vi "Code Compare Tool For Git.vi"() -> ()   [LabVIEW 2016]
doc: "GUI to compare LabVIEW code between currently checked out branch with any other branch or any of its commits"
uses:
  <vilib>/Hampel Software Engineering/Git API/Git API/GIT-api.lvclass
  <vilib>/Hampel Software Engineering/Git API/Git API/GIT-api.lvclass/GIT-api.ctl
  <vilib>/Hampel Software Engineering/Git API/Git API/Controls/GIT-Repository States.ctl
  <vilib>/Utility/miscctls.llb/LVComboBoxStrsAndValuesArrayTypeDef.ctl
  <vilib>/Hampel Software Engineering/Git API/Git API/Accessors/GIT-Set Working Dir.vi
  <userlib>/_OpenG.lib/file/file.llb/Valid Path - Traditional__ogtk.vi
  <userlib>/_OpenG.lib/file/file.llb/File Exists - Scalar__ogtk.vi
  <userlib>/_OpenG.lib/array/array.llb/Delete Elements from 2D Array (String)__ogtk.vi
  <userlib>/_OpenG.lib/array/array.llb/Remove Duplicates from 1D Array (String)__ogtk.vi
  <userlib>/_OpenG.lib/array/array.llb/Search 1D Array (String)__ogtk.vi
  <userlib>/_OpenG.lib/array/array.llb/Remove Duplicates from 1D Array (Path)__ogtk.vi
panel:
  in  "Tab Control":T1(tab)=enum."Main UI"
  in  "All Files Selection":enum8{"False", "True", "Mixed"}(c332)
  in  "Refresh Current Branch":bool
  in  "Commits to Fetch":u32=10 min=1 step=10
  out "No Changes":bool
  in  "Compare Mode":enum32{"With Branch", "With Commit"}(radio)
  out "Commit Details":string
  in  "Commit":string(combo) caption="Recent Commit"
  in  "Stop":bool
  in  "Repository Path":path
  out "Current Branch":string
  in  "Branch":string(combo)="origin/main" caption="Branch to Compare"
  in  "Current Branch Changelist":i32(listbox)=-1
  in  "LabVIEW Compare Filter":bool
  out "Changelist Stats":string
  in  "Compare":bool
  out "Current Branch Status":string
  out "Current Branch Highlight":bool=TRUE
  out "Branch Highlight":bool=TRUE
  out "Commit Highlight":bool
  in  "LabVIEW Compare Options":T2={"VI Attributes"=TRUE, "Front Panel"=TRUE, "FP position/size"=TRUE, "Block Diagram"=TRUE, "BD cosmetic"=TRUE, "BD position/size"=TRUE}
  # "GUI to compare LabVIEW code between currently checked out branch with any other branch or any of its commits.\n\n\n1. Checkout the branch of interest in your system using any method - Git command line, Desktop Git GUI Clients etc.,\n\n2. Specify the local Repository Path.\n\n3. Verify the current branch, its status and select a branch or commit based on the Compare Mode and click on Compare to display the file changes.\n\n4. Double click on a file to initiate LabVIEW code comparison.\n\n5. Once done with required comparisons, exit the tool by closing the window. The tool cleans up the temporary files added during comparison.\n\n\nNote:\n1. This tool uses LabVIEW's VI Comparison Tool which requires LabVIEW Professional Development System.\n2. It is recommended to not use other Git Clients actively when comparing files using this tool to avoid Git command related errors.\n3. It is recommended to commit all changes (working copy) before using this tool for comparison."
  # "This tool uses git diff command to identify the changes. Hence it is recommended to commit all the changes (working copy) to have them considered for comparison.\n\nExample: Identify changes in current branch when comparing with other branch\n\n---A---B---C---D    <== other branch\n               \\\n                 E---F      <== current branch\n\n1. We will need to identify only the file changes introduced by current branch. E and F commits are those changes in the above example (commits after the common ancestor B).\n2. For the identified file changes compare with the other branch (D) to see how it differs. These differences will be our current branch changelist.\n\nWhy only current branch changes?\nIt is most useful to see how the current branch will modify the files when it is getting merged. Best use case for displaying only current branch changelist will be for Pull Request reviews."
  # "*Double click on modified LabVIEW file row to compare\n*Ctrl+Double click on a row to open file"
  # "Type Info:\n \nA - Added                     D - Deleted\nC* - Copied                  R* - Renamed\nM - Modified               T - File type change\nU - File is unmerged   X -  \"unknown\" change type\n\n*Number after C/R indicates the percentage of similarity between original and copied/renamed file"
  # "1. Repository Path - Local repository path (the top level folder with '.git' hidden folder in it). Git API will be initialized for this repository.\n\n2. Current Branch - Currently checked out branch. The status of the current branch is also displayed at top right. Click Refresh button to update the current branch if it is changed in the system or received new changes via Git Pull.\n\n3. Compare Mode - Select the type of comparison. You can compare the current branch with another branch or with a particular commit of a selected branch.\n\nIn branch comparison mode, you can enter the branch name for comparison in Branch to Compare. Remote branches usually start with \"origin/\" and local branches do not have \"origin/\" prefix. The branch's recent commit is displayed in Recent Commit and its details in Commit Details for reference. \n\nIn commit comparison mode, the commits available in the branch selected in Select Branch are listed in Commit to Compare. For the commit selected in Commit to Compare, its details will be displayed in the Commit Details. Use Commits to Fetch to limit the number of commits obtained and improve the loading time.\n\n     Note: Git doesn't maintain information on when the branch is created. So, all the commits of the selected branch will be displayed (all the way up to the very first commit after repository creation). Without a limit, it increases loading time.\n\n4. Compare - Identifies the file changes and Current Branch Changelist table shows the list of all files that are different in the current branch compared to the branch/commit selected.\n\n     Note: The other branch/commit in comparison would have introduced its own changes that are not part of current branch. Those changes will not be displayed.\n\n5. Filter LabVIEW VI and Control Files - Filter files except VI and CTL files. These require LabVIEW to compare but project, library and classes are text files that can be easily reviewed in the desktop Git GUI clients or in Pull Request of Git web services.\n\n6. LabVIEW Compare Options - Options to decide what to compare in the code. Set the required options before initiating code compare.\n\n7. Double click on the file you wish to compare. LabVIEW opens the compare window for the file from the current branch and the file from the other branch/commit (file will be suffixed with TEMP). It may take a while if the VI/CTL have lot of dependencies to load. Having the project pre-opened and opening this tool from that instance may reduce the loading time. Note that the file from the other branch/commit in comparison may be missing its dependent files which may not be available in the current branch or deleted in the current branch commits. This will cause the file to be in a broken state but does not affect the comparison. Another reason for the broken state may be due to the parent library/class not recognizing this new file with the suffix but this as well will not affect the comparison.\n\n     Note: The files from other branch/commit are placed at the same location in the current branch so that the LabVIEW can load the dependencies appropriately.\n\n8. Viewed Status (mixed checkbox) - A tick mark appears for every file compared or opened. Use the mixed checkbox (below the Current Branch Changelist) to control status for all files.\n\n     Note: Viewed status is only a visual aid for tracking and does not have any other function other than that.\n\n9. Panel Close - Stops the tools execution after removing all the new files introduced into the current branch (TEMP files)."
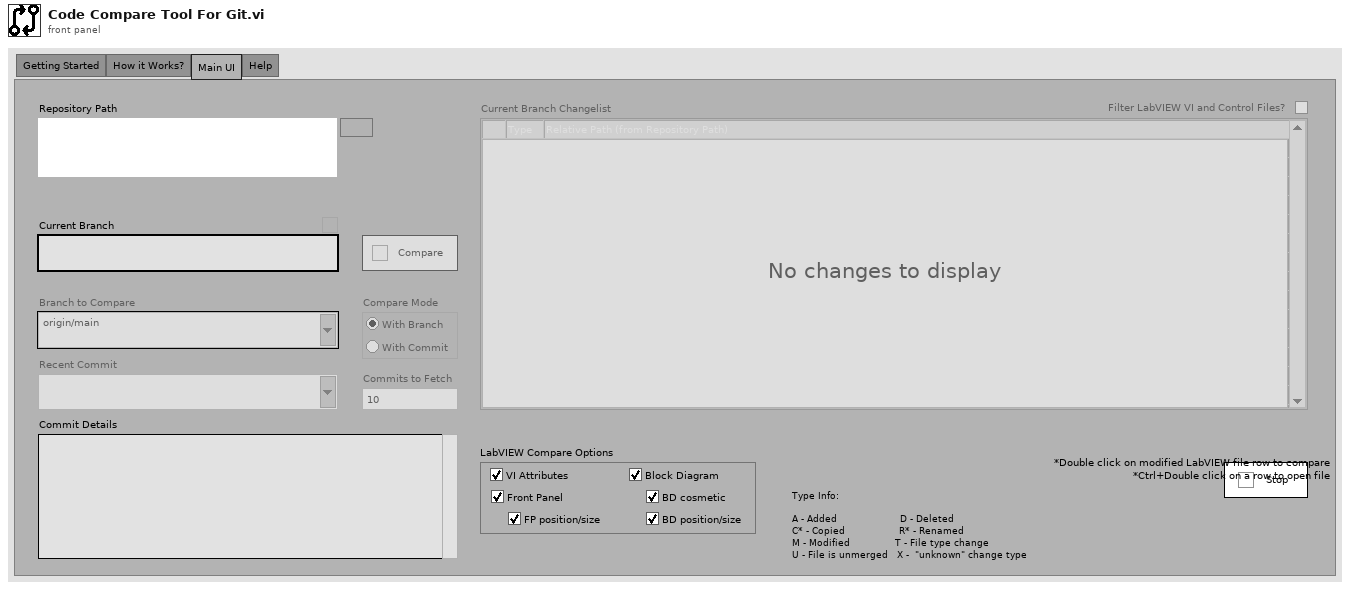
[diagram p1: front panel]
types:
  T1 = enum32{"Getting Started", "How it Works?", "Main UI", "Help"}
  T2 = cluster{"VI Attributes":bool, "Front Panel":bool, "FP position/size":bool, "Block Diagram":bool, "BD cosmetic":bool, "BD position/size":bool}
  T3 = cluster{"Repository Path":path, "Git API Object":refnum<class "GIT-api.lvclass">, "Git API Initialized?":bool, "Current Branch":string, "Compare Mode":enum32{"With Branch", "With Commit"}, "Branch to Compare":string, "Commit to Compare":string, "Commits to Fetch":u32, "Branch/Commit to Compare":string, "Changelist":string[][], "Viewed Files":string[], "Viewed File":string, "LabVIEW Compare Filter":bool, "LabVIEW Compare File Extensions":string[], "File to Open":string, "File to Compare":string, "File to Compare (backup)":path, "File to Compare (other)":path, "LabVIEW Compare Options":cluster{"VI Attributes":bool, "Front Panel":bool, "FP position/size":bool, "Block Diagram":bool, "BD cosmetic":bool, "BD position/size":bool}, "LabVIEW Compare Options Command":string, "Files to Delete":path[]}
  T4 = enum8{"Enabled", "Disabled", "Disabled and Grayed Out"}
  T5 = typedef "GIT-API-for-LabVIEW.lvlib/GIT-api.lvclass/GIT-Repository States.ctl" = enum16{"up-to-date", "behind", "ahead", "diverged", "unpublished", "detached", "unknown"}
  T6 = typedef "LVComboBoxStrsAndValuesArrayTypeDef.ctl" = cluster{"String":string, "Value":string}[]
  T7 = typedef "LVPoint32TypeDef.ctl" = cluster{"Horizontal":i32, "Vertical":i32}
  T8 = typedef "LVRowAndColumnTypeDef.ctl" = cluster{"Row":i32, "Column":i32}
  T9 = enum16{"Left Button", "Center Button", "Right Button", "Window Close"}
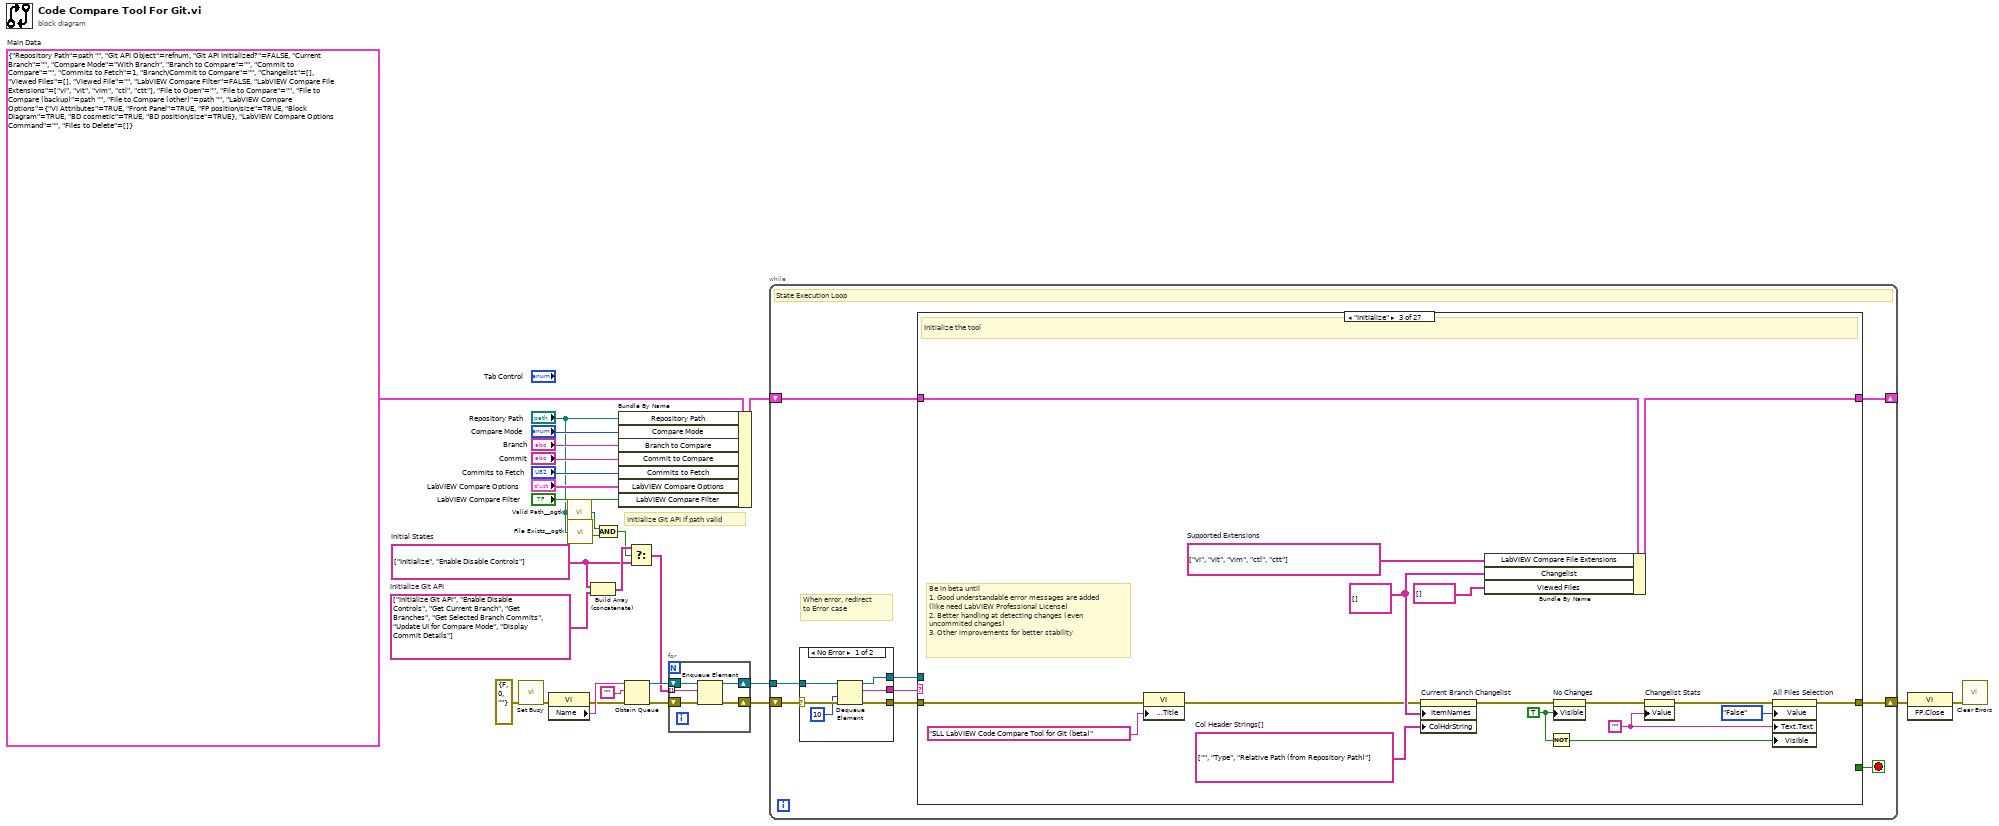
[diagram p0: block diagram]
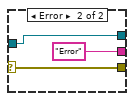
[diagram p2: hidden frame]
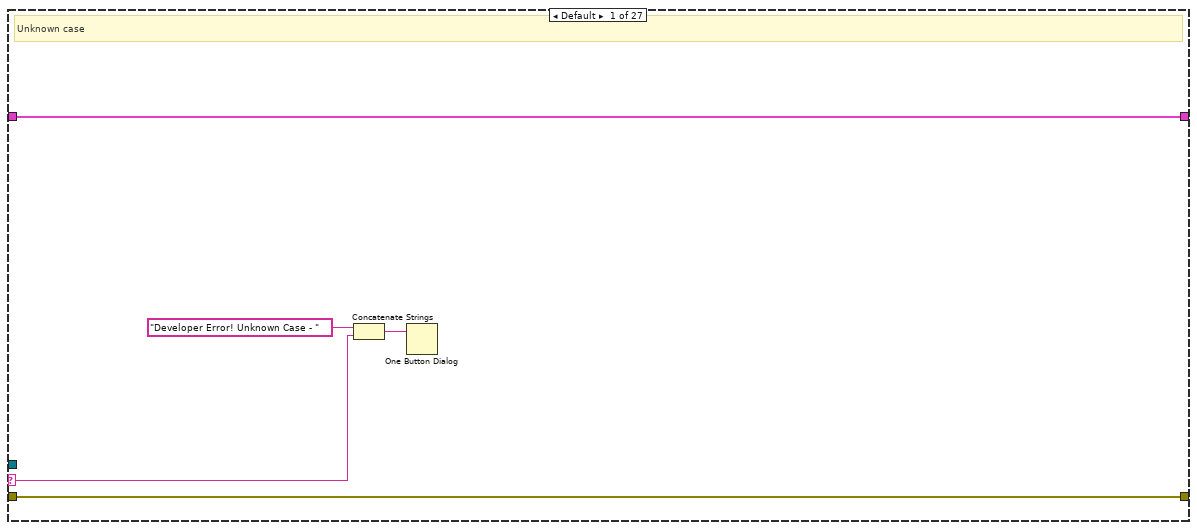
[diagram p3: hidden frame]
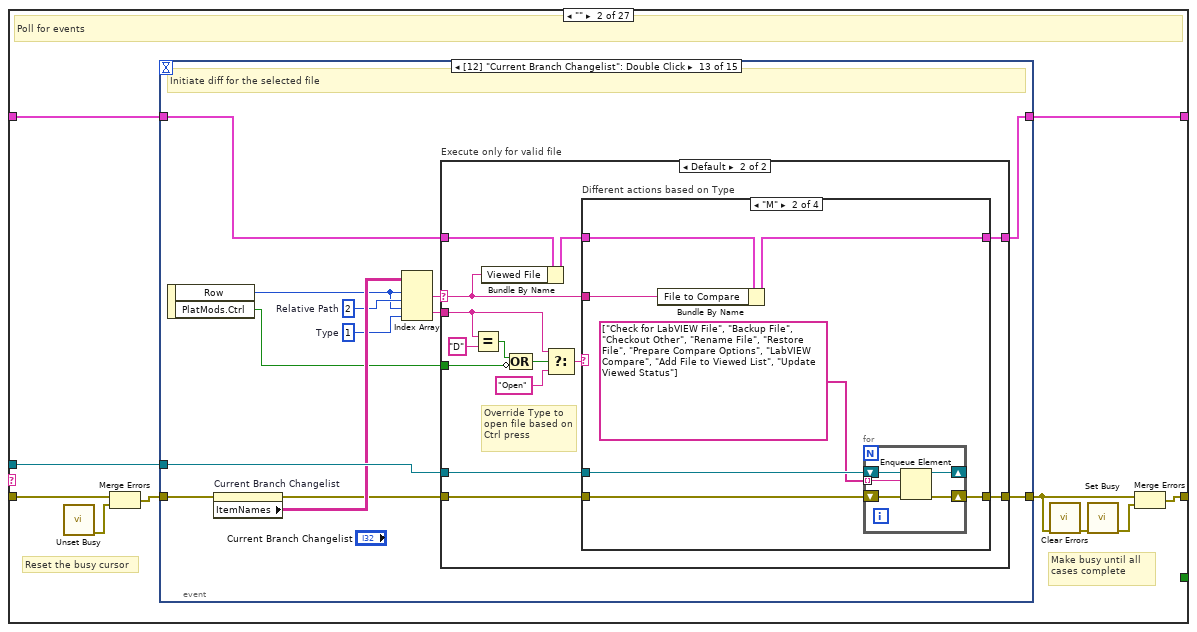
[diagram p4: hidden frame]
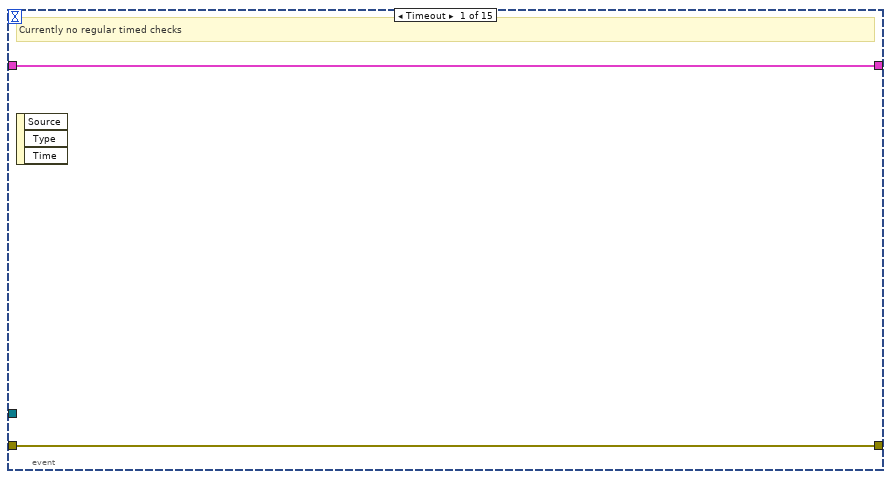
[diagram p5: hidden frame]
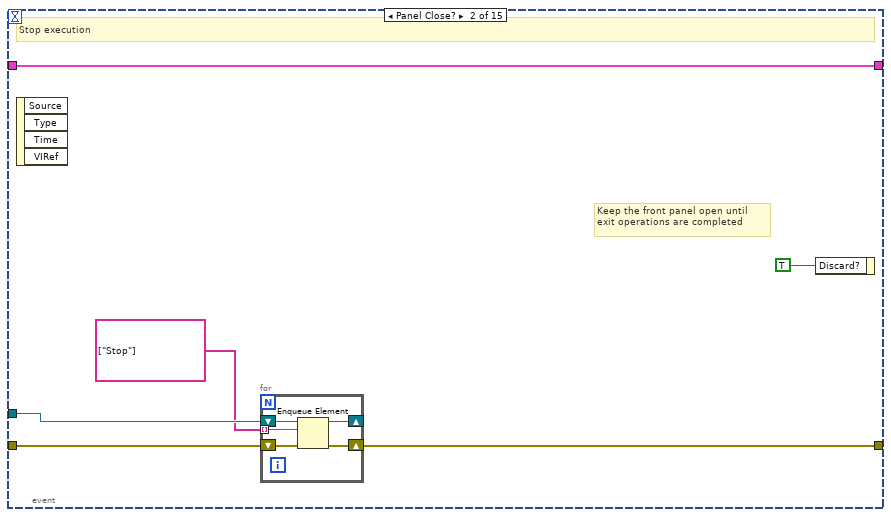
[diagram p6: hidden frame]
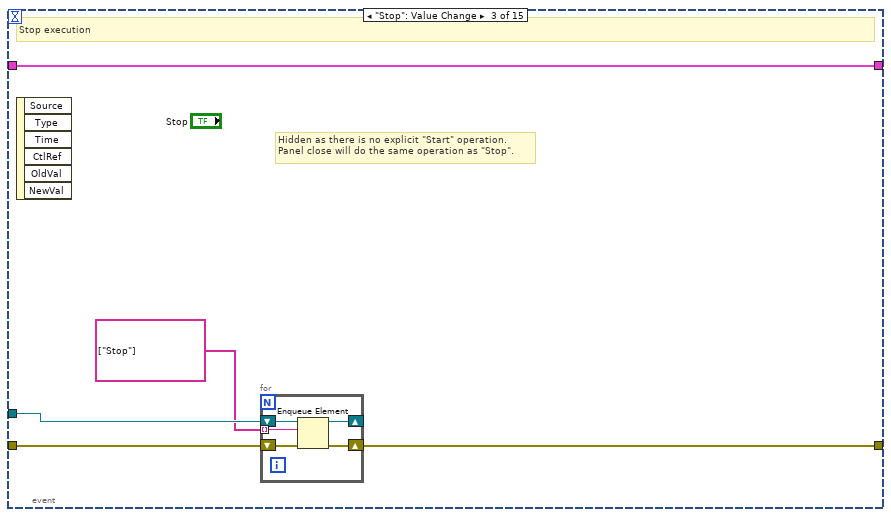
[diagram p7: hidden frame]
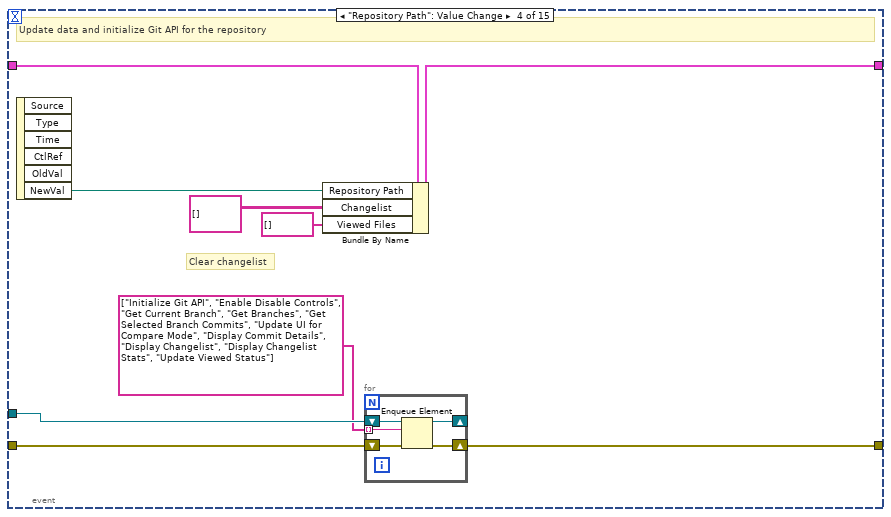
[diagram p8: hidden frame]
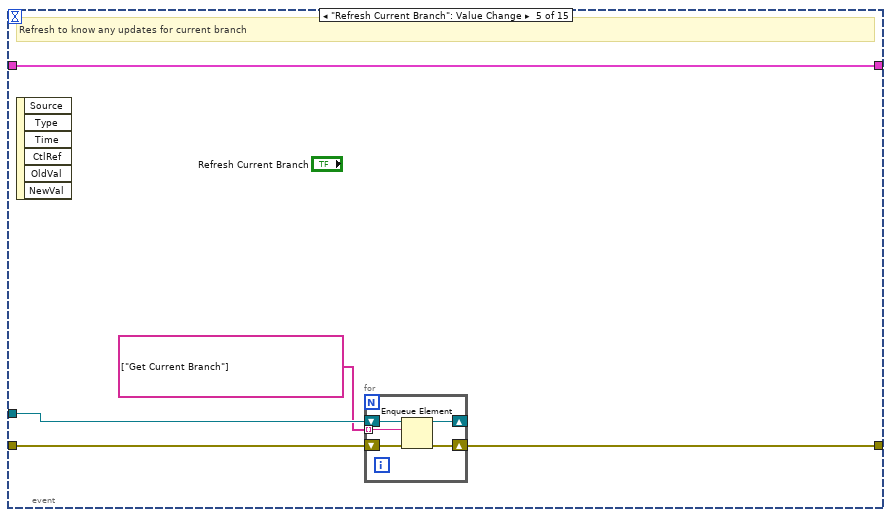
[diagram p9: hidden frame]
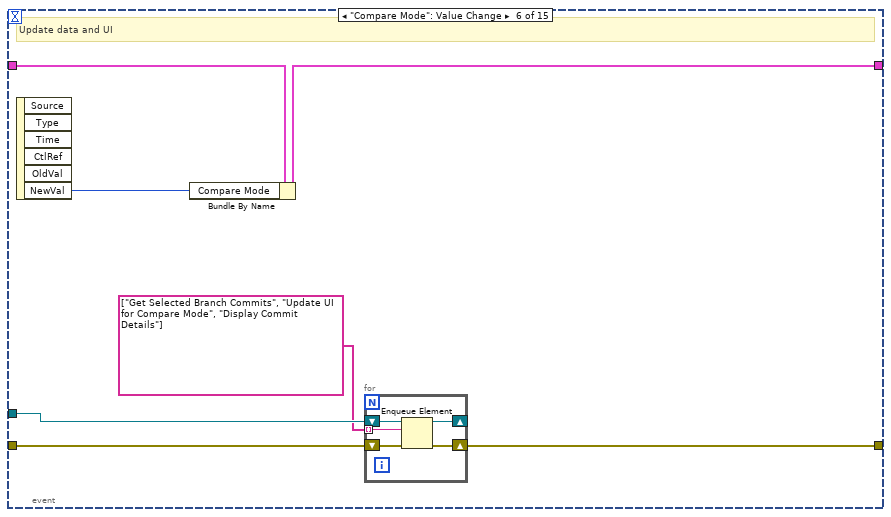
[diagram p10: hidden frame]
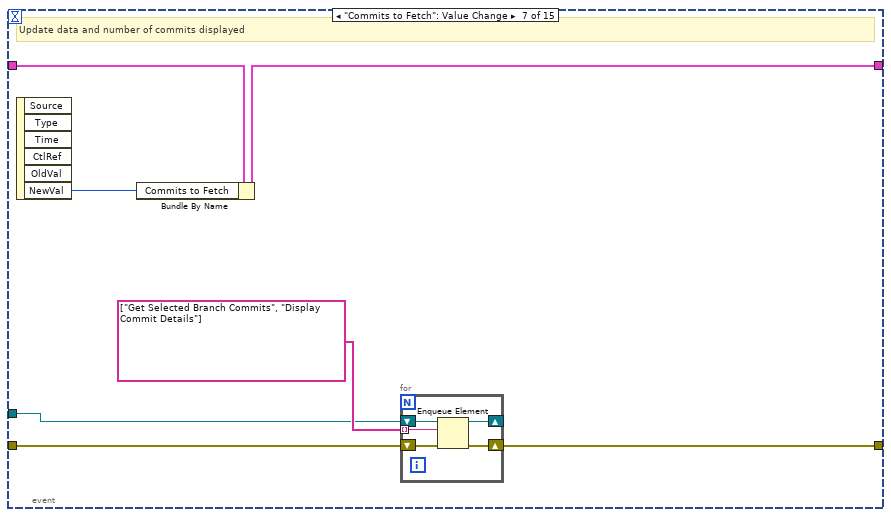
[diagram p11: hidden frame]
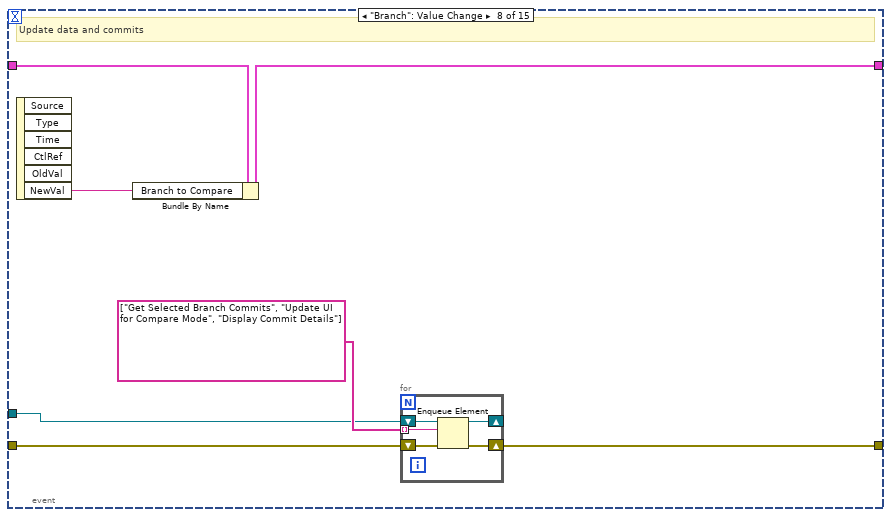
[diagram p12: hidden frame]
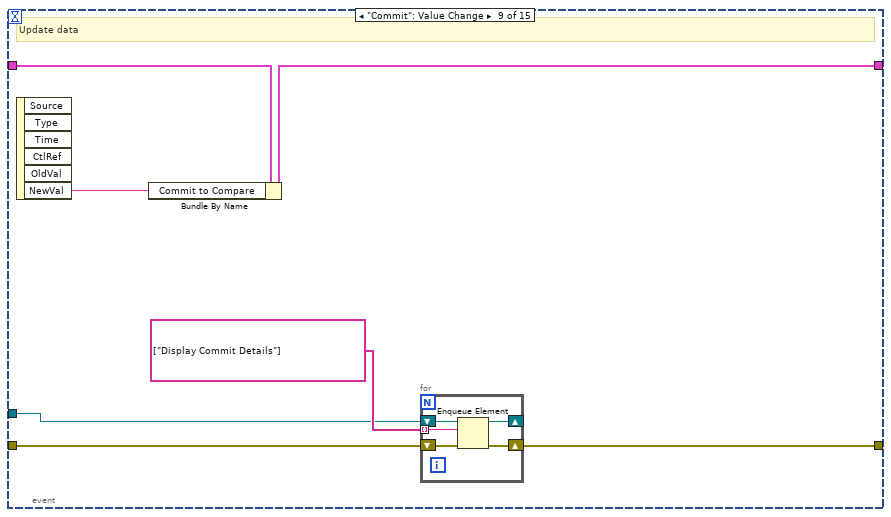
[diagram p13: hidden frame]
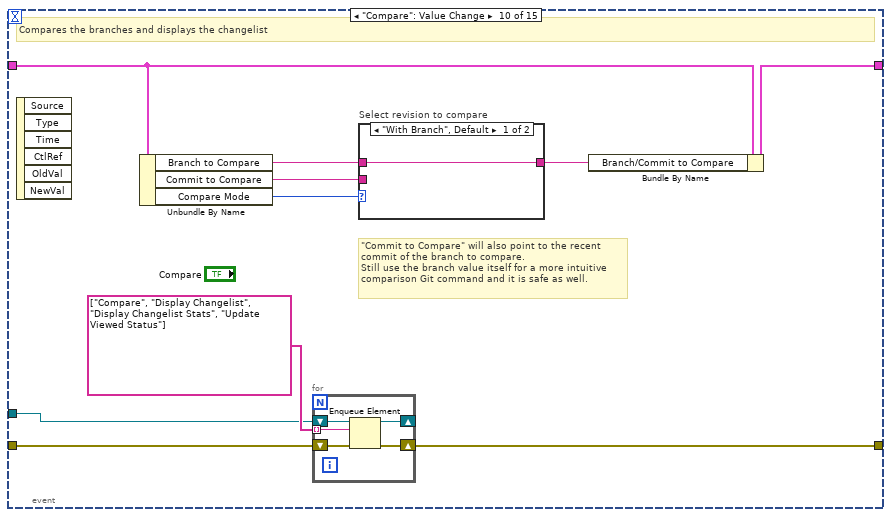
[diagram p14: hidden frame]
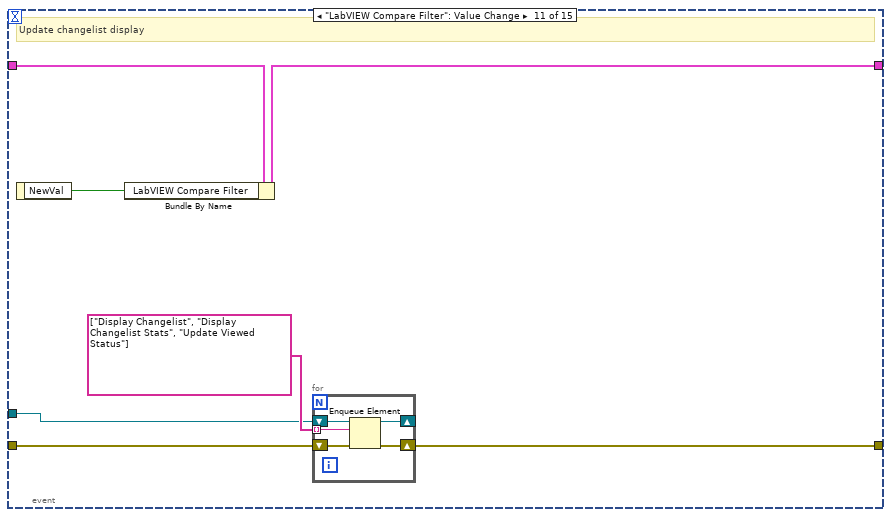
[diagram p16: hidden frame]
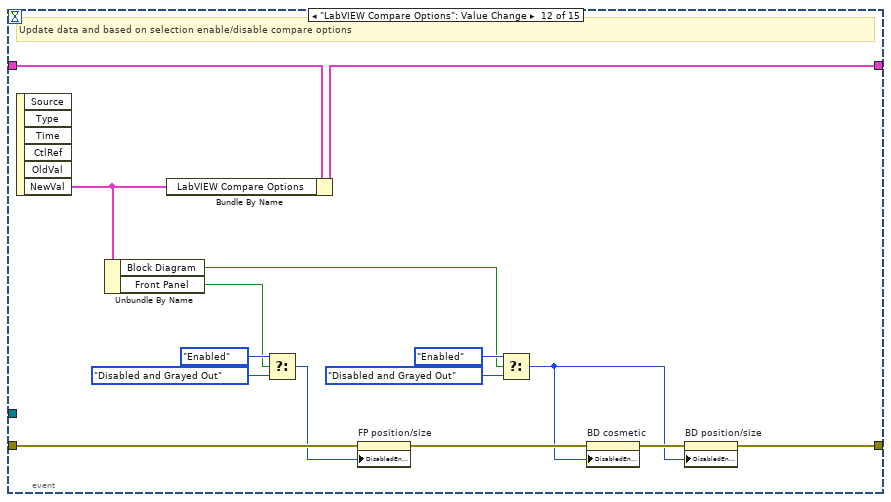
[diagram p17: hidden frame]
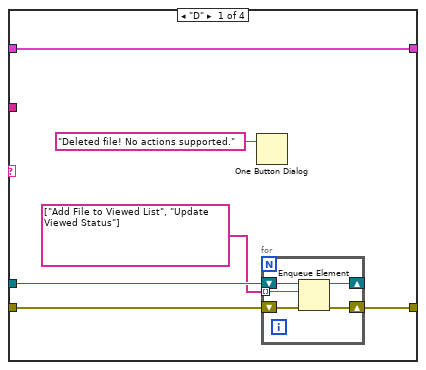
[diagram p19: hidden frame]
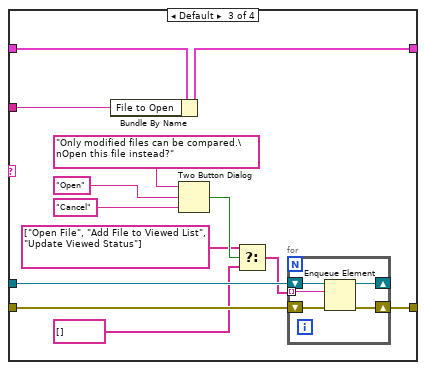
[diagram p20: hidden frame]
diagram:
  w16 = string[] ["Initialize Git API", "Enable Disable Controls", "Get Current Branch", "Get Branches", "Get Selected Branch Commits", "Update UI for Compare Mode", "Display Commit Details"]  # Initialize Git API
  w14 = string[] ["Initialize", "Enable Disable Controls"]  # Initial States
  w24 = T3 {"Repository Path"=path "", "Git API Object"=refnum, "Git API Initialized?"=FALSE, "Current Branch"="", "Compare Mode"=enum."With Branch", "Branch to Compare"="", "Commit to Compare"="", "Commits to Fetch"=1, "Branch/Commit to Compare"="", "Changelist"=[], "Viewed Files"=[], "Viewed File"="", "LabVIEW Compare Filter"=FALSE, "LabVIEW Compare File Extensions"=["vi", "vit", "vim", "ctl", "ctt"], "File to Open"="", "File to Compare"="", "File to Compare (backup)"=path "", "File to Compare (other)"=path "", "LabVIEW Compare Options"={"VI Attributes"=TRUE, "Front Panel"=TRUE, "FP position/size"=TRUE, "Block Diagram"=TRUE, "BD cosmetic"=TRUE, "BD position/size"=TRUE}, "LabVIEW Compare Options Command"="", "Files to Delete"=[]}  # Main Data
  # "Initialize Git API if path valid"
  n1 = call <vilib>:"Set Busy.vi"("error in (no error)"=errorcluster {"status"=FALSE, "code"=0, "source"=""}) -> ("error out"=w7:errorcluster)  [unwired: 9 in, 1 out]
  n2 = property class="VI"(error in=w7) -> (error out=w26:errorcluster, "Name"=w27:string)  [unwired: 1 in, 1 out]
  n3 = call-poly <userlib>:"Valid Path__ogtk.vi"("path"="Repository Path") -> ("valid"=w11:bool)
  n4 = call-poly <userlib>:"File Exists__ogtk.vi"("file path"="Repository Path") -> ("exists"=w12:bool)  [unwired: 6 in, 1 out]
  n5 = Build Array (concatenate)(w14, w16) -> (w15:string[])
  n6 = And(x=w11, y=w12) -> (x .and. y?=w10:bool)
  n7 = Bundle By Name(cluster=w24, "Repository Path"="Repository Path", "Compare Mode"="Compare Mode", "Branch to Compare"="Branch", "Commit to Compare"="Commit", "Commits to Fetch"="Commits to Fetch", "LabVIEW Compare Options"="LabVIEW Compare Options", "LabVIEW Compare Filter"="LabVIEW Compare Filter") -> (w23:T3)
  n8 = Obtain Queue(name (unnamed)=w27, element data type="", error in (no error)=w26) -> (queue out=w20:refnum<queue>, error out=w17:errorcluster)  [unwired: 2 in, 1 out]
  n9 = Select(t=w15, s=w10, f=w14) -> (s? t:f=w13:string[])
  n10 = for {
    tunnel: w13 -> [w29] mode=indexing
    shift-right: [w31] -> w19
    shift-left: w17 -> [w32]
    shift-right: [w28] -> w18
    shift-left: w20 -> [w30]
    n11 = Enqueue Element(queue=w30, element=w29, error in (no error)=w32) -> (queue out=w28:refnum<queue>, error out=w31:errorcluster)  [unwired: 1 in, 1 out]
  }
  n12 = while {
    shift-right: [w33] -> w2
    shift-left: w19 -> [w35]
    tunnel: w18 -> [w36]
    shift-right: [w38] -> _
    shift-left: w23 -> [w37]
    stop <- w39 stop-if-true
    # "When error, redirect to Error case"
    # "State Execution Loop"
    n13 = case shown="No Error" w35 {
      selector: w35 -> [w44 w48]
      tunnel: [w47 "Error" ("element")] -> w41
      tunnel: [w46 w50] -> w40
      tunnel: w36 -> [w45 w50]
      tunnel: [w42 w48] -> w34
      frame No Error {
        n14 = Dequeue Element(queue=w45, timeout in ms (-1)=10, error in (no error)=w44) -> (queue out=w46:refnum<queue>, element=w47:string, error out=w42:errorcluster)  [unwired: 1 out]
      }
      frame Error {
      }
    }
    n15 = case shown="\"Initialize\"" w41 {
      selector: w41 -> [w54 _ _ _ _ _ _ _ _ _ _ _ _ _ _ _ _ _ _ _ _ _ _ _ _ _ _]
      tunnel: w34 -> [w52 w59 w348 w376 w379 w400 w438 w491 w519 w546 w592 w625 w670 w677 w711 w734 w777 w789 w804 w818 w824 w855 w869 w875 w890 w900 w908]
      tunnel: w40 -> [_ w65 _ _ _ _ _ _ _ _ _ _ _ _ _ w731 _ _ _ _ _ _ _ _ w888 w896 w905]
      tunnel: [w52 w61 w355 w364 w383 w409 w448 w478 w524 w545 w557 w624 w655 w677 w697 w730 w776 w793 w797 w822 w830 w855 w867 w874 w889 w897 w901] -> w33
      tunnel: [_ _ _ _ _ _ _ _ _ _ _ _ _ _ _ _ _ _ _ _ _ _ _ _ _ w898 _] -> w39
      tunnel: [w51 w63 w360 w373 w394 w412 w446 w471 w513 w547 w590 w623 w652 w681 w710 w728 w778 w785 w805 w814 w827 w834 w872 w877 w887 w899 w909] -> w38
      tunnel: w37 -> [w51 w64 w361 w375 w394 w413 w447 w472 w514 w547 w570 w623 w652 w682 w710 w729 w778 w786 w805 w815 w827 w835 w872 w877 w887 w899 w909]
      frame Default {
        # "Unknown case"
        n16 = Concatenate Strings("Developer Error! Unknown Case - " ("string"), w54) -> (w53:string)
        n17 = One Button Dialog(message=w53) -> ()  [unwired: 1 in, 1 out]
      }
      frame "" {
        # "Reset the busy cursor"
        # "Make busy until all cases complete"
        # "Poll for events"
        n18 = call <vilib>:"Unset Busy.vi"() -> ("error out"=w60:errorcluster)  [unwired: 11 in]
        n19 = Merge Errors(w59, w60) -> (w58:errorcluster)
        n20 = event shown="[12] \"Current Branch Changelist\": Double Click" {
          selector: _ -> [_ _ _ _ _ _ _ _ _ _ _ _ _ _ _]
          dyn-events: _ -> [_ _ _ _ _ _ _ _ _ _ _ _ _ _ _]
          timeout: _ -> [_ _ _ _ _ _ _ _ _ _ _ _ _ _ _]
          tunnel: w58 -> [w66 w73 w83 w94 w107 w116 w127 w139 w151 w169 w183 w195 w217 w289 w332]
          tunnel: w65 -> [_ w72 w82 w93 w106 w115 w125 w137 w149 w168 w182 _ w214 w301 w333]
          tunnel: [w66 w71 w81 w89 w104 w113 w126 w138 w150 w167 w181 w192 w215 w302 w324] -> w57
          tunnel: w64 -> [w67 w70 w80 w97 w103 w119 w131 w143 w155 w166 w180 w204 w206 w300 w329]
          tunnel: [w67 w70 w80 w96 w103 w118 w130 w142 w154 w165 w179 w203 w216 w303 w328] -> w63
          event Timeout {
            # "Currently no regular timed checks"
            n21 = event-data() -> ()  [unwired: 1 in, 3 out]
          }
          event Panel Close? {
            # "Keep the front panel open until exit operations are completed"
            # "Stop execution"
            n22 = event-data() -> ()  [unwired: 1 in, 4 out]
            n23 = for {
              tunnel: string[] ["Stop"] -> [w75] mode=indexing
              shift-right: [w77] -> w71
              shift-left: w73 -> [w78]
              shift-right: [w74] -> _
              shift-left: w72 -> [w76]
              n24 = Enqueue Element(queue=w76, element=w75, error in (no error)=w78) -> (queue out=w74:refnum<queue>, error out=w77:errorcluster)  [unwired: 1 in, 1 out]
            }
            n25 = event-data("Discard?"=TRUE) -> ()  [unwired: 1 in, 1 out]
          }
          event "Stop": Value Change {
            # "Hidden as there is no explicit \"Start\" operation.\nPanel close will do the same operation as \"Stop\"."
            # "Stop execution"
            n26 = event-data() -> ()  [unwired: 1 in, 6 out]
            n27 = for {
              tunnel: string[] ["Stop"] -> [w85] mode=indexing
              shift-right: [w87] -> w81
              shift-left: w83 -> [w88]
              shift-right: [w84] -> _
              shift-left: w82 -> [w86]
              n28 = Enqueue Element(queue=w86, element=w85, error in (no error)=w88) -> (queue out=w84:refnum<queue>, error out=w87:errorcluster)  [unwired: 1 in, 1 out]
            }
          }
          event "Repository Path": Value Change {
            # "Clear changelist"
            # "Update data and initialize Git API for the repository"
            n29 = event-data() -> ("NewVal"=w95:path)  [unwired: 1 in, 5 out]
            n30 = Bundle By Name(cluster=w97, "Repository Path"=w95, "Changelist"=string[][] [] ("Item Names"), "Viewed Files"=string[] []) -> (w96:T3)
            n31 = for {
              tunnel: string[] ["Initialize Git API", "Enable Disable Controls", "Get Current Branch", "Get Branches", "Get Selected Branch Commits", "Update UI for Compare Mode", "Display Commit Details", "Display Changelist", "Display Changelist Stats", "Update Viewed Status"] -> [w99] mode=indexing
              shift-right: [w101] -> w89
              shift-left: w94 -> [w102]
              shift-right: [w98] -> _
              shift-left: w93 -> [w100]
              n32 = Enqueue Element(queue=w100, element=w99, error in (no error)=w102) -> (queue out=w98:refnum<queue>, error out=w101:errorcluster)  [unwired: 1 in, 1 out]
            }
          }
          event "Refresh Current Branch": Value Change {
            # "Refresh to know any updates for current branch"
            n33 = event-data() -> ()  [unwired: 1 in, 6 out]
            n34 = for {
              tunnel: string[] ["Get Current Branch"] -> [w109] mode=indexing
              shift-right: [w111] -> w104
              shift-left: w107 -> [w112]
              shift-right: [w108] -> _
              shift-left: w106 -> [w110]
              n35 = Enqueue Element(queue=w110, element=w109, error in (no error)=w112) -> (queue out=w108:refnum<queue>, error out=w111:errorcluster)  [unwired: 1 in, 1 out]
            }
          }
          event "Compare Mode": Value Change {
            # "Update data and UI"
            n36 = event-data() -> ("NewVal"=w117:enum32{"With Branch", "With Commit"})  [unwired: 1 in, 5 out]
            n37 = Bundle By Name(cluster=w119, "Compare Mode"=w117) -> (w118:T3)
            n38 = for {
              tunnel: string[] ["Get Selected Branch Commits", "Update UI for Compare Mode", "Display Commit Details"] -> [w121] mode=indexing
              shift-right: [w123] -> w113
              shift-left: w116 -> [w124]
              shift-right: [w120] -> _
              shift-left: w115 -> [w122]
              n39 = Enqueue Element(queue=w122, element=w121, error in (no error)=w124) -> (queue out=w120:refnum<queue>, error out=w123:errorcluster)  [unwired: 1 in, 1 out]
            }
          }
          event "Commits to Fetch": Value Change {
            # "Update data and number of commits displayed"
            n40 = event-data() -> ("NewVal"=w129:u32)  [unwired: 1 in, 5 out]
            n41 = Bundle By Name(cluster=w131, "Commits to Fetch"=w129) -> (w130:T3)
            n42 = for {
              tunnel: string[] ["Get Selected Branch Commits", "Display Commit Details"] -> [w133] mode=indexing
              shift-right: [w135] -> w126
              shift-left: w127 -> [w136]
              shift-right: [w132] -> _
              shift-left: w125 -> [w134]
              n43 = Enqueue Element(queue=w134, element=w133, error in (no error)=w136) -> (queue out=w132:refnum<queue>, error out=w135:errorcluster)  [unwired: 1 in, 1 out]
            }
          }
          event "Branch": Value Change {
            # "Update data and commits"
            n44 = event-data() -> ("NewVal"=w141:string)  [unwired: 1 in, 5 out]
            n45 = Bundle By Name(cluster=w143, "Branch to Compare"=w141) -> (w142:T3)
            n46 = for {
              tunnel: string[] ["Get Selected Branch Commits", "Update UI for Compare Mode", "Display Commit Details"] -> [w145] mode=indexing
              shift-right: [w147] -> w138
              shift-left: w139 -> [w148]
              shift-right: [w144] -> _
              shift-left: w137 -> [w146]
              n47 = Enqueue Element(queue=w146, element=w145, error in (no error)=w148) -> (queue out=w144:refnum<queue>, error out=w147:errorcluster)  [unwired: 1 in, 1 out]
            }
          }
          event "Commit": Value Change {
            # "Update data"
            n48 = event-data() -> ("NewVal"=w153:string)  [unwired: 1 in, 5 out]
            n49 = Bundle By Name(cluster=w155, "Commit to Compare"=w153) -> (w154:T3)
            n50 = for {
              tunnel: string[] ["Display Commit Details"] -> [w157] mode=indexing
              shift-right: [w159] -> w150
              shift-left: w151 -> [w160]
              shift-right: [w156] -> _
              shift-left: w149 -> [w158]
              n51 = Enqueue Element(queue=w158, element=w157, error in (no error)=w160) -> (queue out=w156:refnum<queue>, error out=w159:errorcluster)  [unwired: 1 in, 1 out]
            }
          }
          event "Compare": Value Change {
            # "\"Commit to Compare\" will also point to the recent commit of the branch to compare.\nStill use the branch value itself for a more intuitive comparison Git command and it is safe as well."
            # "Compares the branches and displays the changelist"
            n52 = event-data() -> ()  [unwired: 1 in, 6 out]
            n53 = Unbundle By Name(w166) -> ("Branch to Compare"=w162:string, "Commit to Compare"=w163:string, "Compare Mode"=w164:enum32{"With Branch", "With Commit"})
            n54 = for {
              tunnel: string[] ["Compare", "Display Changelist", "Display Changelist Stats", "Update Viewed Status"] -> [w174] mode=indexing
              shift-right: [w176] -> w167
              shift-left: w169 -> [w177]
              shift-right: [w173] -> _
              shift-left: w168 -> [w175]
              n55 = Enqueue Element(queue=w175, element=w174, error in (no error)=w177) -> (queue out=w173:refnum<queue>, error out=w176:errorcluster)  [unwired: 1 in, 1 out]
            }
            n56 = case "Select revision to compare" shown="\"With Branch\", Default" w164 {
              tunnel: w163 -> [_ w172]
              tunnel: w162 -> [w171 _]
              tunnel: [w171 w172] -> w161
              frame "With Branch", Default {
              }
              frame "With Commit" {
              }
            }
            n57 = Bundle By Name(cluster=w166, "Branch/Commit to Compare"=w161) -> (w165:T3)
          }
          event "LabVIEW Compare Filter": Value Change {
            # "Update changelist display"
            n58 = event-data() -> ("NewVal"=w178:bool)  [unwired: 1 in]
            n59 = Bundle By Name(cluster=w180, "LabVIEW Compare Filter"=w178) -> (w179:T3)
            n60 = for {
              tunnel: string[] ["Display Changelist", "Display Changelist Stats", "Update Viewed Status"] -> [w186] mode=indexing
              shift-right: [w188] -> w181
              shift-left: w183 -> [w189]
              shift-right: [w185] -> _
              shift-left: w182 -> [w187]
              n61 = Enqueue Element(queue=w187, element=w186, error in (no error)=w189) -> (queue out=w185:refnum<queue>, error out=w188:errorcluster)  [unwired: 1 in, 1 out]
            }
          }
          event "LabVIEW Compare Options": Value Change {
            # "Update data and based on selection enable/disable compare options"
            n62 = event-data() -> ("NewVal"=w202:T2)  [unwired: 1 in, 5 out]
            n63 = Unbundle By Name(w202) -> ("Block Diagram"=w197:bool, "Front Panel"=w196:bool)
            n64 = Bundle By Name(cluster=w204, "LabVIEW Compare Options"=w202) -> (w203:T3)
            n65 = Select(t=T4."Enabled" ("Disabled"), s=w196, f=T4."Disabled and Grayed Out" ("Disabled")) -> (s? t:f=w193:T4)
            n66 = property on="FP position/size" class="Bool (strict)"(error in=w195, "DisabledEnum"=w193) -> (error out=w194:errorcluster)  [unwired: 1 in, 1 out]
            n67 = Select(t=T4."Enabled" ("Disabled"), s=w197, f=T4."Disabled and Grayed Out" ("Disabled")) -> (s? t:f=w190:T4)
            n68 = property on="BD cosmetic" class="Bool (strict)"(error in=w194, "DisabledEnum"=w190) -> (error out=w191:errorcluster)  [unwired: 1 in, 1 out]
            n69 = property on="BD position/size" class="Bool (strict)"(error in=w191, "DisabledEnum"=w190) -> (error out=w192:errorcluster)  [unwired: 1 in, 1 out]
          }
          event "Current Branch Changelist": Double Click {
            w208 = 1  # Type
            w212 = 2  # Relative Path
            # "Initiate diff for the selected file"
            n70 = event-data() -> ("Row"=w209:i32, "PlatMods.Ctrl"=w205:bool)  [unwired: 1 in]
            n71 = property on="Current Branch Changelist" class="MCListbox (strict)"(error in=w217) -> (error out=w210:errorcluster, "ItemNames"=w213:string[][])  [unwired: 1 in, 1 out]
            n72 = Index Array(array=w213, index (row) #1=w209, index (col) #1=w212, index (row) #2=w209, index (col) #2=w208) -> (element #1=w211:string, element #2=w207:string)
            n73 = case "Execute only for valid file" shown="Default" w211 {
              selector: w211 -> [_ w229]
              tunnel: w206 -> [w218 w228]
              tunnel: [w218 w233] -> w216
              tunnel: [w219 w232] -> w215
              tunnel: w214 -> [_ w231]
              tunnel: w210 -> [w219 w230]
              tunnel: w207 -> [_ w224]
              tunnel: w205 -> [_ w221]
              frame "" {
              }
              frame Default {
                # "Override Type to open file based on Ctrl press"
                n74 = Equal?(x=w224, y="D") -> (x = y?=w222:bool)
                n75 = Bundle By Name(cluster=w228, "Viewed File"=w229) -> (w227:T3)
                n76 = Compound Arithmetic op=OR(w222, invert w221) -> (w220:bool)
                n77 = Select(t=w224, s=w220, f="Open") -> (s? t:f=w225:string)
                n78 = case "Different actions based on Type" shown="\"M\"" w225 {
                  tunnel: w227 -> [w239 w251 w269 w281]
                  tunnel: [w239 w250 w268 w280] -> w233
                  tunnel: [w236 w249 w267 w279] -> w232
                  tunnel: w231 -> [w235 w248 w266 w278]
                  tunnel: w229 -> [_ w247 w265 w277]
                  tunnel: w230 -> [w237 w246 w264 w276]
                  frame "D" {
                    n79 = One Button Dialog(message="Deleted file! No actions supported." ("format string")) -> ()  [unwired: 1 in, 1 out]
                    n80 = for {
                      tunnel: string[] ["Add File to Viewed List", "Update Viewed Status"] -> [w241] mode=indexing
                      shift-right: [w243] -> w236
                      shift-left: w237 -> [w244]
                      shift-right: [w240] -> _
                      shift-left: w235 -> [w242]
                      n81 = Enqueue Element(queue=w242, element=w241, error in (no error)=w244) -> (queue out=w240:refnum<queue>, error out=w243:errorcluster)  [unwired: 1 in, 1 out]
                    }
                  }
                  frame "M" {
                    n82 = Bundle By Name(cluster=w251, "File to Compare"=w247) -> (w250:T3)
                    n83 = for {
                      tunnel: string[] ["Check for LabVIEW File", "Backup File", "Checkout Other", "Rename File", "Restore File", "Prepare Compare Options", "LabVIEW Compare", "Add File to Viewed List", "Update Viewed Status"] -> [w253] mode=indexing
                      shift-right: [w255] -> w249
                      shift-left: w246 -> [w256]
                      shift-right: [w252] -> _
                      shift-left: w248 -> [w254]
                      n84 = Enqueue Element(queue=w254, element=w253, error in (no error)=w256) -> (queue out=w252:refnum<queue>, error out=w255:errorcluster)  [unwired: 1 in, 1 out]
                    }
                  }
                  frame Default {
                    n85 = Bundle By Name(cluster=w269, "File to Open"=w265) -> (w268:T3)
                    n86 = Two Button Dialog(message="Only modified files can be compared.\nOpen this file instead?", 1:"Cancel" ("F button name (\"Cancel\")"), 2:"Open" ("T button name (\"OK\")")) -> (T button?=w260:bool)
                    n87 = Select(t=string[] ["Open File", "Add File to Viewed List", "Update Viewed Status"], s=w260, f=string[] []) -> (s? t:f=w259:string[])
                    n88 = for {
                      tunnel: w259 -> [w271] mode=indexing
                      shift-right: [w273] -> w267
                      shift-left: w264 -> [w274]
                      shift-right: [w270] -> _
                      shift-left: w266 -> [w272]
                      n89 = Enqueue Element(queue=w272, element=w271, error in (no error)=w274) -> (queue out=w270:refnum<queue>, error out=w273:errorcluster)  [unwired: 1 in, 1 out]
                    }
                  }
                  frame "Open" {
                    n90 = Bundle By Name(cluster=w281, "File to Open"=w277) -> (w280:T3)
                    n91 = for {
                      tunnel: string[] ["Open File", "Add File to Viewed List", "Update Viewed Status"] -> [w283] mode=indexing
                      shift-right: [w285] -> w279
                      shift-left: w276 -> [w286]
                      shift-right: [w282] -> _
                      shift-left: w278 -> [w284]
                      n92 = Enqueue Element(queue=w284, element=w283, error in (no error)=w286) -> (queue out=w282:refnum<queue>, error out=w285:errorcluster)  [unwired: 1 in, 1 out]
                    }
                  }
                }
              }
            }
          }
          event "Current Branch Changelist": Mouse Up {
            w294 = 2  # Relative Path
            # "Check for mouse click on symbol and take action"
            n93 = event-data() -> ("Coords"=w297:T7)  [unwired: 1 in]
            n94 = property on="Current Branch Changelist" class="MCListbox (strict)"(error in=w289) -> (error out=w288:errorcluster, "ItemNames"=w287:string[][])  [unwired: 1 in, 1 out]
            n95 = Unbundle By Name(w300) -> ("Viewed Files"=w298:string[])
            n96 = invoke on="Current Branch Changelist" class="MCListbox (strict)" method="Point To Row Column"(error in=w288, "Point"=w297) -> (error out=w299:errorcluster, "CellPosition"=w296:T8, "InGlyph"=w292:bool)  [unwired: 5 in, 4 out]
            n97 = Unbundle By Name(w296) -> ("Row"=w295:i32)
            n98 = Index Array(array=w287, index (row)=w295, index (col)=w294) -> (element=w293:string)
            n99 = Empty String/Path?(string/path=w293) -> (empty?=w291:bool)
            n100 = Compound Arithmetic op=AND(invert w291, w292) -> (w290:bool)
            n101 = case "Execute only if clicked on symbol for valid file" shown="True" w290 {
              tunnel: w300 -> [w304 w315]
              tunnel: [w304 w309] -> w303
              tunnel: [w305 w318] -> w302
              tunnel: w301 -> [_ w317]
              tunnel: w299 -> [w305 w316]
              tunnel: w298 -> [_ w308]
              tunnel: w293 -> [_ w311]
              frame False {
              }
              frame True {
                # "Toggle View Status.\nIf not added already, add.\nIf already added, remove."
                n102 = Search 1D Array(1D array=w308, element=w311) -> (index of element=w307:i32)  [unwired: 1 in]
                n103 = Less Than 0?(x=w307) -> (x < 0?=w314:bool)
                n104 = Insert Into Array(array=w308, new element=w311) -> (w313:string[])  [unwired: 1 in]
                n105 = Delete From Array(array=w308, index=w307) -> (array with subset deleted=w306:string[])  [unwired: 1 in, 1 out]
                n106 = Select(t=w313, s=w314, f=w306) -> (s? t:f=w312:string[])
                n107 = for {
                  tunnel: string[] ["Update Viewed Status"] -> [w320] mode=indexing
                  shift-right: [w322] -> w318
                  shift-left: w316 -> [w323]
                  shift-right: [w319] -> _
                  shift-left: w317 -> [w321]
                  n108 = Enqueue Element(queue=w321, element=w320, error in (no error)=w323) -> (queue out=w319:refnum<queue>, error out=w322:errorcluster)  [unwired: 1 in, 1 out]
                }
                n109 = Bundle By Name(cluster=w315, "Viewed Files"=w312) -> (w309:T3)
              }
            }
          }
          event "All Files Selection": Value Change {
            # "Setting the expected value explicitly to avoid confusion with the default state transitions"
            # "Select all or Deselect all files"
            n110 = event-data() -> ("OldVal"=w334:enum8{"False", "True", "Mixed"})  [unwired: 1 in]
            n111 = Unbundle By Name(w329) -> ("Changelist"=w330:string[][])
            n112 = case shown="\"False\"" w334 {
              tunnel: [w340 w345] -> w331
              tunnel: w330 -> [w343 _]
              tunnel: [w341 string[] [] ("Viewed Files")] -> w327
              frame "False" {
                w340 = enum8{"False", "True", "Mixed"}."True"  # Select All
                w342 = 2  # Relative Path
                # "Set Viewed for all files"
                n113 = Index Array(array=w343, index (col)=w342) -> (element=w341:string[])  [unwired: 1 in]
              }
              frame "True", "Mixed" {
                w345 = enum8{"False", "True", "Mixed"}."False"  # Deselect All
                # "Clear Viewed for all files"
              }
            }
            n114 = property on="All Files Selection" class="MixedCheckbox (strict)"(error in=w332, "Value"=w331) -> (error out=w325:errorcluster)  [unwired: 1 in, 1 out]
            n115 = Bundle By Name(cluster=w329, "Viewed Files"=w327) -> (w328:T3)
            n116 = for {
              tunnel: string[] ["Update Viewed Status"] -> [w336] mode=indexing
              shift-right: [w338] -> w324
              shift-left: w325 -> [w339]
              shift-right: [w335] -> _
              shift-left: w333 -> [w337]
              n117 = Enqueue Element(queue=w337, element=w336, error in (no error)=w339) -> (queue out=w335:refnum<queue>, error out=w338:errorcluster)  [unwired: 1 in, 1 out]
            }
          }
        }
        n118 = call <vilib>:"Clear Errors.vi"("error in (no error)"=w57) -> ("error out"=w56:errorcluster)  [unwired: 5 in, 1 out]
        n119 = call <vilib>:"Set Busy.vi"("error in (no error)"=w56) -> ("error out"=w62:errorcluster)  [unwired: 9 in, 1 out]
        n120 = Merge Errors(w57, w62) -> (w61:errorcluster)
      }
      frame "Initialize" {
        w349 = string[] ["vi", "vit", "vim", "ctl", "ctt"]  # Supported Extensions
        w353 = TRUE ("Visible")
        w350 = ""
        w359 = string[][] [] ("Changelist")
        w362 = string[] ["", "Type", "Relative Path (from Repository Path)"]  # Col Header Strings[]
        # "Be in beta until\n1. Good understandable error messages are added (like need LabVIEW Professional License)\n2. Better handling at detecting changes (even uncommited changes)\n3. Other improvements for better stability"
        # "Initialize the tool"
        n121 = property class="VI"(error in=w348, "Front Panel.Title"="SLL LabVIEW Code Compare Tool for Git (beta)" ("string")) -> (error out=w347:errorcluster)  [unwired: 1 in, 1 out]
        n122 = property on="Current Branch Changelist" class="MCListbox (strict)"(error in=w347, "ItemNames"=w359, "ColHdrString"=w362) -> (error out=w357:errorcluster)  [unwired: 1 in, 1 out]
        n123 = Bundle By Name(cluster=w361, "LabVIEW Compare File Extensions"=w349, "Changelist"=w359, "Viewed Files"=string[] []) -> (w360:T3)
        n124 = Not(x=w353) -> (.not. x?=w352:bool)
        n125 = property on="No Changes" class="Bool (strict)"(error in=w357, "Visible"=w353) -> (error out=w358:errorcluster)  [unwired: 1 in, 1 out]
        n126 = property on="Changelist Stats" class="Str"(error in=w358, "Value"=w350) -> (error out=w351:errorcluster)  [unwired: 1 in, 1 out]
        n127 = property on="All Files Selection" class="MixedCheckbox (strict)"(error in=w351, "Value"=enum8{"False", "True", "Mixed"}."False" ("All Files Selection"), "Text.Text"=w350, "Visible"=w352) -> (error out=w355:errorcluster)  [unwired: 1 in, 1 out]
      }
      frame "Initialize Git API" {
        # "Update the actual top level repository path (will be skipped if the repo was not initialized)"
        # "Initializes the Git API"
        n128 = Unbundle By Name(w375) -> ("Repository Path"=w372:path)
        n129 = call <vilib>:"GIT-Create API.vi"("error in"=w376) -> ("error out"=w371:errorcluster, "git-api out"=w369:refnum<class "GIT-api.lvclass">)  [unwired: 9 in]
        n130 = call <vilib>:"GIT-Repository Top Level.vi"("error in"=w371, "Current Path"=w372, "git-api in"=w369) -> ("error out"=w368:errorcluster, "Repo Top Level Path"=w363:path, "git-api out"=w370:refnum<class "GIT-api.lvclass">)  [unwired: 6 in]
        n131 = property class="Git-API"(reference=w370, error in=w368, "Accessors:Working Dir"=w363) -> (reference out=w374:refnum<class "GIT-api.lvclass">, error out=w365:errorcluster)
        n132 = Unbundle By Name(w365) -> ("status"=w367:bool)
        n133 = property on="Repository Path" class="Path"(error in=w365, "Value"=w363) -> (error out=w364:errorcluster)  [unwired: 1 in, 1 out]
        n134 = Not(x=w367) -> (.not. x?=w366:bool)
        n135 = Bundle By Name(cluster=w375, "Git API Object"=w374, "Git API Initialized?"=w366, "Repository Path"=w363) -> (w373:T3)
      }
      frame "Enable Disable Controls" {
        # "Enable or disable controls based on Git API initialized or not"
        n136 = Unbundle By Name(w394) -> ("Git API Initialized?"=w393:bool)
        n137 = Select(t=T4."Enabled" ("Disabled"), s=w393, f=T4."Disabled and Grayed Out" ("Disabled")) -> (s? t:f=w378:T4)
        n138 = property on="Refresh Current Branch" class="Bool"(error in=w379, "DisabledEnum"=w378) -> (error out=w386:errorcluster)  [unwired: 1 in, 1 out]
        n139 = property on="Compare" class="Bool"(error in=w379, "DisabledEnum"=w378) -> (error out=w380:errorcluster)  [unwired: 1 in, 1 out]
        n140 = property on="Current Branch Changelist" class="MCListbox (strict)"(error in=w379, "DisabledEnum"=w378) -> (error out=w381:errorcluster)  [unwired: 1 in, 1 out]
        n141 = property on="Branch" class="CmbBox"(error in=w380, "DisabledEnum"=w378) -> (error out=w390:errorcluster)  [unwired: 1 in, 1 out]
        n142 = property on="All Files Selection" class="MixedCheckbox (strict)"(error in=w381, "DisabledEnum"=w378) -> (error out=w382:errorcluster)  [unwired: 1 in, 1 out]
        n143 = property on="Commit" class="CmbBox"(error in=w390, "DisabledEnum"=w378) -> (error out=w388:errorcluster)  [unwired: 1 in, 1 out]
        n144 = property on="Changelist Stats" class="Str"(error in=w382, "DisabledEnum"=w378) -> (error out=w377:errorcluster)  [unwired: 1 in, 1 out]
        n145 = property on="Compare Mode" class="RadioBtnsControl (strict)"(error in=w388, "DisabledEnum"=w378) -> (error out=w387:errorcluster)  [unwired: 1 in, 1 out]
        n146 = property on="No Changes" class="Bool (strict)"(error in=w377, "DisabledEnum"=w378) -> (error out=w389:errorcluster)  [unwired: 1 in, 1 out]
        n147 = property on="Commits to Fetch" class="DigNum (strict)"(error in=w387, "DisabledEnum"=w378) -> (error out=w385:errorcluster)  [unwired: 1 in, 1 out]
        n148 = property on="LabVIEW Compare Filter" class="Bool (strict)"(error in=w389, "DisabledEnum"=w378) -> (error out=w384:errorcluster)  [unwired: 1 in, 1 out]
        n149 = Merge Errors(w386, w385, w384) -> (w383:errorcluster)
      }
      frame "Get Current Branch" {
        # "Fetch updates from all remotes"
        # "Identify the currently checked out branch and its status and update the UI control"
        n150 = Unbundle By Name(w413) -> ("Git API Object"=w401:refnum<class "GIT-api.lvclass">)
        n151 = call <vilib>:"GIT-Fetch.vi"("param"="--all", "error in"=w400, "git-api in"=w401) -> ("error out"=w406:errorcluster, "git-api out"=w407:refnum<class "GIT-api.lvclass">)  [unwired: 6 in, 1 out]
        n152 = call <vilib>:"GIT-Repository Status.vi"("error in"=w406, "git-api in"=w407) -> ("error out"=w415:errorcluster, "State"=w398:T5, "git-api out"=w414:refnum<class "GIT-api.lvclass">)  [unwired: 6 in, 1 out]
        n153 = call <vilib>:"GIT-Current Branch.vi"("error in"=w415, "git-api in"=w414) -> ("error out"=w399:errorcluster, "current branch"=w402:string)  [unwired: 7 in, 1 out]
        n154 = Equal?(x=GIT-Repository_States."detached", y=w398) -> (x = y?=w403:bool)
        n155 = Select(t="HEAD", s=w403, f=w402) -> (s? t:f=w397:string)
        "Current Branch" <- w397
        n156 = Format Into String(format string="%s", error in=w399, w398) -> (resulting string=→"Current Branch Status":string, error out=w395:errorcluster)  [unwired: 1 in]
        n157 = case "Color for quick identification" shown="\"up-to-date\"" w398 {
          tunnel: [u32 32768 u32 16711680 u32 16860 u32 16744448 u32 16777222 u32 7171459 u32 16711680] -> w408
          frame "up-to-date" {
          }
          frame "behind" {
          }
          frame "ahead" {
          }
          frame "diverged" {
          }
          frame "unpublished" {
          }
          frame "detached" {
          }
          frame "unknown" {
          }
        }
        n158 = Bundle By Name(cluster=w413, "Current Branch"=w397) -> (w412:T3)
        n159 = property on="Current Branch Status" class="Str"(error in=w395, "Text.TextColor"=w408) -> (error out=w409:errorcluster)  [unwired: 1 in, 1 out]
      }
      frame "Get Branches" {
        w428 = 0  # Branch Name List
        w433 = string[][] []
        w432 = "%s" ("format string")
        # "Combine local and remote branches"
        # "List Local branches"
        # "List Remote branches\nNote: All remote branches usually start with origin/ unless renamed"
        # "Reset if previous value not found"
        # "Get all local and remote branches and update UI control"
        n160 = Unbundle By Name(w447) -> ("Git API Object"=w436:refnum<class "GIT-api.lvclass">)
        n161 = call <vilib>:"GIT-Branch.vi"("error in"=w438, "git-api in"=w436) -> ("error out"=w437:errorcluster, "std out"=w429:string, "git-api out"=w430:refnum<class "GIT-api.lvclass">)  [unwired: 7 in]
        n162 = call <vilib>:"GIT-Branch.vi"("param"="-r", "error in"=w437, "git-api in"=w430) -> ("error out"=w440:errorcluster, "std out"=w431:string)  [unwired: 6 in, 1 out]
        n163 = Spreadsheet String To Array(format string=w432, spreadsheet string=w429, array type (2D Dbl)=w433) -> (array=w450:string[][])  [unwired: 1 in]
        n164 = Spreadsheet String To Array(format string=w432, spreadsheet string=w431, array type (2D Dbl)=w433) -> (array=w434:string[][])  [unwired: 1 in]
        n165 = Index Array(array=w450, index (col)=w428) -> (element=w435:string[])  [unwired: 1 in]
        n166 = Index Array(array=w434, index (col)=w428) -> (element=w423:string[])  [unwired: 1 in]
        n167 = for "Remove current branch pointer" {
          tunnel: w435 -> [w459] mode=indexing
          tunnel: [w455] -> w427 mode=indexing
          tunnel: [w454] -> w451 mode=indexing
          n168 = Search and Replace String(input string=w459, search string="*", replace string="") -> (result string=w456:string, error out=w454:errorcluster)  [unwired: 5 in, 2 out]
          n169 = call <vilib>:"Trim Whitespace.vi"("string"=w456) -> ("trimmed string"=w455:string)  [unwired: 1 in]
        }
        n170 = for {
          tunnel: [w453] -> w424 mode=indexing
          tunnel: w423 -> [w452] mode=indexing
          n171 = call <vilib>:"Trim Whitespace.vi"("string"=w452) -> ("trimmed string"=w453:string)  [unwired: 1 in]
        }
        n172 = Build Array (concatenate)(w427, w424) -> (w426:string[])
        n173 = Merge Errors(w440, w451) -> (w425:errorcluster)
        n174 = property on="Branch" class="CmbBox"(error in=w425, "Strings[]"=w426) -> (error out=w449:errorcluster, "Value"=w442:string)  [unwired: 1 in, 1 out]
        n175 = Search 1D Array(1D array=w426, element=w442) -> (index of element=w445:i32)  [unwired: 1 in]
        n176 = Greater Or Equal To 0?(x=w445) -> (x >= 0?=w444:bool)
        n177 = Select(t=w442, s=w444, f="") -> (s? t:f=w441:string)
        n178 = property on="Branch" class="CmbBox"(error in=w449, "Value"=w441) -> (error out=w448:errorcluster)  [unwired: 1 in, 1 out]
        n179 = Bundle By Name(cluster=w447, "Branch to Compare"=w441) -> (w446:T3)
      }
      frame "Get Selected Branch Commits" {
        # "Limit how many commits to fetch. More commits will take long time. For branch comparison, recent 1 commit is enough."
        # "Note: For long list of commits its better only read the Hash and Subject as it is faster due to less contents.\nThen based on selection we can get the full commit details on demand."
        # "Hash is Value\nSubject is String"
        # "Reset if previous value not found"
        # "To avoid coercion dot"
        # "find separator here"
        # "Use the same separator used during the \"git log\" format options"
        # "Get only Hash and Subject"
        # "Get required commits from selected branch and update UI control"
        n180 = Unbundle By Name(w472) -> ("Branch to Compare"=w469:string, "Commits to Fetch"=w462:u32, "Compare Mode"=w464:enum32{"With Branch", "With Commit"}, "Git API Object"=w490:refnum<class "GIT-api.lvclass">)
        n181 = Equal?(x=w464, y=enum32{"With Branch", "With Commit"}."With Commit") -> (x = y?=w465:bool)
        n182 = Select(t=w462, s=w465, f=u32 1) -> (s? t:f=w461:u32)
        n183 = Format Value(format string=" -%u", value (0)=w461) -> (output string=w466:string)  [unwired: 1 in]
        n184 = Concatenate Strings(w469, " --format=\"%H|%s\"" ("string"), w466) -> (w487:string)
        n185 = case "Only for valid branch" shown="Default" w469 {
          tunnel: w491 -> [w493 w499]
          tunnel: w490 -> [_ w498]
          tunnel: [w493 w497] -> w489
          tunnel: w487 -> [_ w496]
          tunnel: ["" ("std out") w494] -> w468
          frame "" {
          }
          frame Default {
            n186 = call <vilib>:"GIT-Log.vi"("param"=w496, "error in"=w499, "git-api in"=w498) -> ("error out"=w497:errorcluster, "std out"=w495:string)  [unwired: 6 in, 1 out]
            n187 = call <vilib>:"Trim Whitespace.vi"("string"=w495) -> ("trimmed string"=w494:string)  [unwired: 1 in]
          }
        }
        n188 = Spreadsheet String To Array(delimiter (Tab)="|", format string="%s", spreadsheet string=w468, array type (2D Dbl)=string[][] []) -> (array=w483:string[][])
        n189 = for "For every commit" {
          tunnel: w483 -> [w504] mode=indexing
          tunnel: [w501] -> w481 mode=indexing
          tunnel: [w500] -> w477 mode=indexing
          n190 = Index Array(array=w504) -> (element #1=w500:string, element #2=w502:string)  [unwired: 2 in]
          n191 = Bundle By Name(cluster=cluster{"String":string, "Value":string} {"String"="", "Value"=""}, "Value"=w500, "String"=w502) -> (w501:cluster{"String":string, "Value":string})
        }
        n192 = Insert Into Array(array=T6 [] ("Strings And Values []"), new element=w481) -> (w480:T6)  [unwired: 1 in]
        n193 = property on="Commit" class="CmbBox"(error in=w489, "Strings And Values[]"=w480) -> (error out=w479:errorcluster, "Value"=w474:string)  [unwired: 1 in, 1 out]
        n194 = Search 1D Array(1D array=w477, element=w474) -> (index of element=w476:i32)  [unwired: 1 in]
        n195 = Greater Or Equal To 0?(x=w476) -> (x >= 0?=w475:bool)
        n196 = Select(t=w474, s=w475, f="") -> (s? t:f=w470:string)
        n197 = property on="Commit" class="CmbBox"(error in=w479, "Value"=w470) -> (error out=w478:errorcluster)  [unwired: 1 in, 1 out]
        n198 = Bundle By Name(cluster=w472, "Commit to Compare"=w470) -> (w471:T3)
      }
      frame "Update UI for Compare Mode" {
        # "First value is the recent commit"
        # "Based on compare mode selected, update the UI display"
        n199 = property on="Commit" class="CmbBox"(error in=w519) -> (error out=w523:errorcluster, "Value"=w518:string, "Strings And Values[]"=w517:T6)  [unwired: 1 in, 1 out]
        n200 = Unbundle By Name(w514) -> ("Compare Mode"=w525:enum32{"With Branch", "With Commit"})
        n201 = Index Array(array=w517) -> (element=w516:cluster{"String":string, "Value":string})  [unwired: 1 in]
        n202 = Unbundle By Name(w516) -> ("Value"=w515:string)
        n203 = case "Update Captions and State" shown="\"With Branch\", Default" w525 {
          tunnel: [w533 w541] -> w520
          tunnel: [w532 w540] -> w522
          tunnel: [T4."Disabled and Grayed Out" ("Disabled") T4."Enabled" ("Disabled")] -> w505
          tunnel: w518 -> [_ w538]
          tunnel: [w530 w538] -> w510
          tunnel: w515 -> [w530 _]
          tunnel: [w529 w537] -> w512
          tunnel: [w528 w536] -> w511
          tunnel: [TRUE FALSE] -> w509
          tunnel: [FALSE TRUE] -> w508
          frame "With Branch", Default {
            w528 = "Recent commit of branch to compare"  # Tip Strip
            w529 = "The branch to compare the current branch against"  # Tip Strip
            w532 = "Recent Commit"  # Caption
            w533 = "Branch to Compare"  # Caption
            # "For branch, use recent commit"
          }
          frame "With Commit" {
            w536 = "Selected branch commits"  # Tip Strip
            w537 = "Select branch to list its commits"  # Tip Strip
            w540 = "Commit to Compare"  # Caption
            w541 = "Select Branch"  # Caption
          }
        }
        "Branch Highlight" <- w509
        "Commit Highlight" <- w508
        n204 = property on="Commit" class="CmbBox"(error in=w523, "Caption.Text"=w522, "TipStrip"=w511, "DisabledEnum"=w505, "Value"=w510) -> (error out=w506:errorcluster)  [unwired: 1 in, 1 out]
        n205 = property on="Commits to Fetch" class="DigNum (strict)"(error in=w506, "DisabledEnum"=w505) -> (error out=w521:errorcluster)  [unwired: 1 in, 1 out]
        n206 = property on="Branch" class="CmbBox"(error in=w521, "Caption.Text"=w520, "TipStrip"=w512) -> (error out=w524:errorcluster)  [unwired: 1 in, 1 out]
        n207 = Bundle By Name(cluster=w514, "Commit to Compare"=w510) -> (w513:T3)
        "Current Branch Highlight" <- TRUE ("Current Branch Highlight")
      }
      frame "Display Commit Details" {
        # "Display more details about the selected commit"
        n208 = Unbundle By Name(w547) -> ("Git API Object"=w544:refnum<class "GIT-api.lvclass">, "Commit to Compare"=w543:string)
        n209 = case "Display only for non-empty commit" shown="Default" w543 {
          selector: w543 -> [_ w552]
          tunnel: w546 -> [w549 w555]
          tunnel: [w549 w554] -> w545
          tunnel: w544 -> [_ w553]
          tunnel: ["" ("Commit Info") w551] -> w542
          frame "" {
          }
          frame Default {
            n210 = call <vilib>:"GIT-Commit Info.vi"("Format String"="Commit Hash: %H\nCommitter: %cN <%cE>\nDate: %cd (%cr)\n\n%s\n%b", "error in"=w555, "Commit"=w552, "git-api in"=w553) -> ("error out"=w554:errorcluster, "Commit Info"=w551:string)  [unwired: 5 in, 1 out]
          }
        }
        "Commit Details" <- w542
      }
      frame "Compare" {
        w593 = 2  # Renamed/Copied Path
        w564 = 0  # Type
        w572 = string[][] []
        w571 = "%s" ("format string")
        w581 = 1  # Relative Path
        w569 = " --name-status" ("string")
        # "Reset Viewed status"
        # "For Viewed column"
        # "If we have the renamed/copied path, we need to use that. Since this column can be fully empty, not using auto indexing as empty column array will stop For loop execution"
        # "For renames and copies, this column holds the current relative path"
        # "Example: Identify changes in branch2 when comparing with branch1\n\n---A---B---C---D  <== branch1\n                 \\\n                   E---F        <== branch2\n\ngit diff branch1...branch2\n=> diff between B & F (includes E & F changes, B is common ancestor)\n\ngit diff branch1..branch2\n=> diff between D & F (includes E, F, C & D changes)\n\nWe wanted diff between D & F only but without any changes of C & D that is unrelated to branch2 (like new files/changes only available in branch1 which is not in interest for branch2). So get branch2's changes using 3 dot diff (file paths) and get the actual diff of those file(s) using 2 dot diff (change types)."
        # "Filter files that are not available in two dot diff. Remember we wanted two dot diff only but used 3 dot diff to identify current branch's changes."
        # "Change slash to backslash for path (Windows recognizable format)"
        # "Two dot diff alone will list unwanted changes from other branch/commit that is not in relation to current branch's changes.\nSo use three dot diff to identify the current branch's changes and get the actual change type from two dot diff."
        # "Identifies changes introduced in current branch compared to the other branch/commit"
        n211 = Unbundle By Name(w570) -> ("Branch/Commit to Compare"=w575:string, "Current Branch"=w573:string, "Git API Object"=w591:refnum<class "GIT-api.lvclass">)
        n212 = Concatenate Strings(w575, "..", w573, w569) -> (w588:string)
        n213 = Concatenate Strings(w575, "...", w573, w569) -> (w585:string)
        n214 = call <vilib>:"GIT-Diff.vi"("param"=w588, "error in"=w592, "git-api in"=w591) -> ("error out"=w587:errorcluster, "std out"=w568:string, "git-api out"=w586:refnum<class "GIT-api.lvclass">)  [unwired: 6 in]
        n215 = call <vilib>:"GIT-Diff.vi"("param"=w585, "error in"=w587, "git-api in"=w586) -> ("error out"=w566:errorcluster, "std out"=w567:string)  [unwired: 6 in, 1 out]
        n216 = Spreadsheet String To Array(format string=w571, spreadsheet string=w568, array type (2D Dbl)=w572) -> (array=w584:string[][])  [unwired: 1 in]
        n217 = Spreadsheet String To Array(format string=w571, spreadsheet string=w567, array type (2D Dbl)=w572) -> (array=w563:string[][])  [unwired: 1 in]
        n218 = Index Array(array=w584, index (col) #1=w564, index (col) #2=w581, index (col) #3=w593) -> (element #1=w583:string[], element #2=w582:string[], element #3=w561:string[])  [unwired: 3 in]
        n219 = Index Array(array=w563, index (col) #1=w564, index (col) #2=w581, index (col) #3=w593) -> (element #2=w580:string[], element #3=w562:string[])  [unwired: 3 in, 1 out]
        n220 = for "Format and create changelist" {
          tunnel: w580 -> [w607] mode=indexing
          tunnel: [w612] -> w579 mode=indexing if=w595
          tunnel: w582 -> [w603]
          tunnel: w583 -> [w611]
          tunnel: [w610] -> w578 mode=indexing if=w595
          tunnel: [w608] -> w565 mode=indexing
          tunnel: w562 -> [w606]
          tunnel: w561 -> [w602]
          tunnel: [""] -> w559 mode=indexing if=w595
          i -> [w599]
          w598 = TRUE  # replace all?
          n221 = Index Array(array=w606, index=w599) -> (element=w600:string)
          n222 = Empty String/Path?(string/path=w600) -> (empty?=w604:bool)
          n223 = Select(t=w603, s=w604, f=w602) -> (s? t:f=w601:string[])
          n224 = Select(t=w607, s=w604, f=w600) -> (s? t:f=w605:string)
          n225 = Search 1D Array(1D array=w601, element=w605) -> (index of element=w609:i32)  [unwired: 1 in]
          n226 = Search and Replace String(replace all?=w598, input string=w605, search string="/", replace string="\\" ("replace string (\"\")")) -> (result string=w612:string, error out=w608:errorcluster)  [unwired: 4 in, 2 out]
          n227 = Greater Or Equal To 0?(x=w609) -> (x >= 0?=w595:bool)
          n228 = Index Array(array=w611, index=w609) -> (element=w610:string)
        }
        n229 = Build Array(w559, w578, w579) -> (w577:string[][])
        n230 = Merge Errors(w566, w565) -> (w556:errorcluster)
        n231 = Transpose 2D Array(2D array=w577) -> (transposed array=w576:string[][])
        n232 = property on="All Files Selection" class="MixedCheckbox (strict)"(error in=w556, "Value"=enum8{"False", "True", "Mixed"}."False" ("All Files Selection")) -> (error out=w557:errorcluster)  [unwired: 1 in, 1 out]
        n233 = Bundle By Name(cluster=w570, "Changelist"=w576, "Viewed Files"=string[] []) -> (w590:T3)
      }
      frame "Display Changelist" {
        # "Clear the viewed stats"
        # "Highlight only for no changes during comparison to provide UI feedback.\nFor filtering, it is understood that there aren't such files to display."
        # "Show the changelist in UI"
        n234 = Unbundle By Name(w623) -> ("LabVIEW Compare Filter"=w622:bool, "Changelist"=w620:string[][], "LabVIEW Compare File Extensions"=w617:string[])
        n235 = Empty Array?(array=w620) -> (empty?=w614:bool)
        n236 = case "Filter files for LabVIEW?" shown="True" w622 {
          tunnel: w620 -> [w631 w637]
          tunnel: [w631 w634] -> w621
          tunnel: [_ w633] -> w618
          tunnel: w617 -> [_ w632]
          frame False {
          }
          frame True {
            w638 = 2  # Relative Path
            # "Delete other files"
            n237 = Index Array(array=w637, index (col)=w638) -> (element=w639:string[])  [unwired: 1 in]
            n238 = for "Identify index for files other than LabVIEW" {
              tunnel: w639 -> [w645] mode=indexing
              tunnel: [w644] -> w635 mode=indexing if=w640
              tunnel: [w647] -> w633 mode=indexing
              tunnel: w632 -> [w643]
              i -> [w644]
              n239 = String To Path(string=w645) -> (path=w646:path)
              n240 = call <vilib>:"Get File Extension.vi"("file"=w646) -> ("error out"=w647:errorcluster, "lowercase file extension"=w642:string)  [unwired: 6 in, 3 out]
              n241 = Search 1D Array(1D array=w643, element=w642) -> (index of element=w641:i32)  [unwired: 1 in]
              n242 = Less Than 0?(x=w641) -> (x < 0?=w640:bool)
            }
            n243 = call-poly <userlib>:"Delete Elements from Array__ogtk.vi"("delete (rows or columns)"=enum16{"rows", "columns"}."rows", "indices"=w635, "array"=w637) -> ("array w/ subset deleted"=w634:string[][])  [unwired: 7 in, 1 out]
          }
        }
        n244 = property on="No Changes" class="Bool (strict)"(error in=w625, "Visible"=w614) -> (error out=w626:errorcluster)  [unwired: 1 in, 1 out]
        n245 = Not(x=w614) -> (.not. x?=w616:bool)
        n246 = property on="All Files Selection" class="MixedCheckbox (strict)"(error in=w626, "Visible"=w616) -> (error out=w613:errorcluster)  [unwired: 1 in, 1 out]
        n247 = case "Empty changelist?" shown="True" w614 {
          tunnel: w613 -> [w627 w630]
          tunnel: [w627 w629] -> w615
          frame False {
          }
          frame True {
            n248 = property on="All Files Selection" class="MixedCheckbox (strict)"(error in=w630, "Text.Text"="") -> (error out=w629:errorcluster)  [unwired: 1 in, 1 out]
          }
        }
        n249 = Merge Errors(w615, w618) -> (w619:errorcluster)
        n250 = property on="Current Branch Changelist" class="MCListbox (strict)"(error in=w619, "ItemNames"=w621) -> (error out=w624:errorcluster)  [unwired: 1 in, 1 out]
      }
      frame "Display Changelist Stats" {
        w669 = 1  # Type
        # "Show the changelist stats"
        n251 = Unbundle By Name(w652) -> ("LabVIEW Compare Filter"=w651:bool)
        n252 = property on="Current Branch Changelist" class="MCListbox (strict)"(error in=w670) -> (error out=w655:errorcluster, "ItemNames"=w654:string[][])  [unwired: 1 in, 1 out]
        n253 = Index Array(array=w654, index (col)=w669) -> (element=w659:string[])  [unwired: 1 in]
        n254 = Empty Array?(array=w659) -> (empty?=w658:bool)
        n255 = Select(t="(Filtered files - %u." ("string (\"\")"), s=w651, f="(Total files - %u." ("string (\"\")")) -> (s? t:f=w648:string)
        n256 = Array Size(array=w659) -> (size(s)=w667:i32)
        n257 = call-poly <userlib>:"Remove Duplicates from 1D Array__ogtk.vi"("Input Array"=w659) -> ("Output Array"=w668:string[])  [unwired: 1 out]
        n258 = for "Get Count for each Type" {
          tunnel: w668 -> [w674] mode=indexing
          tunnel: w659 -> [w676]
          tunnel: [w671] -> w664 mode=indexing
          n259 = call-poly <userlib>:"Search Array__ogtk.vi"("Array"=w676, "Element Data"=w674) -> ("Indices of Elements"=w675:i32[])  [unwired: 7 in]
          n260 = Array Size(array=w675) -> (size(s)=w672:i32)
          n261 = Format Value(string ("")=w674, format string=" - %u", value (0)=w672) -> (output string=w671:string)
        }
        n262 = Format Value(format string=w648, value (0)=w667) -> (output string=w662:string)  [unwired: 1 in]
        n263 = Array To Spreadsheet String(delimiter (Tab)=", ", array=w664, 3:"%s" ("spreadsheet string")) -> (spreadsheet string=w663:string)
        n264 = call <vilib>:"Trim Whitespace.vi"("string"=w663) -> ("trimmed string"=w660:string)  [unwired: 1 in]
        n265 = Format Value(string ("")=w662, format string=" %s)", value (0)=w660) -> (output string=w657:string)
        n266 = Select(t="", s=w658, f=w657) -> (s? t:f=→"Changelist Stats":string)
      }
      frame "Add File to Viewed List" {
        # "Add to Viewed paths if not added already"
        # "Update Viewed Paths List"
        n267 = Unbundle By Name(w682) -> ("Viewed Files"=w680:string[], "Viewed File"=w679:string)
        n268 = Insert Into Array(array=w680, new element=w679) -> (w683:string[])  [unwired: 1 in]
        n269 = Search 1D Array(1D array=w680, element=w679) -> (index of element=w685:i32)  [unwired: 1 in]
        n270 = Less Than 0?(x=w685) -> (x < 0?=w684:bool)
        n271 = Select(t=w683, s=w684, f=w680) -> (s? t:f=w678:string[])
        n272 = Bundle By Name(cluster=w682, "Viewed Files"=w678) -> (w681:T3)
      }
      frame "Update Viewed Status" {
        w695 = 2  # Relative Path
        # "Set the value and  viewed stats"
        # "Sorting both array's will make the order same for easier comparison"
        # "Update Viewed Status for all files"
        n273 = property on="Current Branch Changelist" class="MCListbox (strict)"(error in=w711) -> (error out=w708:errorcluster, "ItemNames"=w689:string[][])  [unwired: 1 in, 1 out]
        n274 = Unbundle By Name(w710) -> ("Changelist"=w688:string[][], "Viewed Files"=w693:string[])
        n275 = Index Array(array=w688, index (col)=w695) -> (element=w694:string[])  [unwired: 1 in]
        n276 = Index Array(array=w689, index (col)=w695) -> (element=w709:string[])  [unwired: 1 in]
        n277 = Empty Array?(array=w688) -> (empty?=w687:bool)
        n278 = for "Get Viewed for each File" {
          tunnel: w709 -> [w725] mode=indexing
          tunnel: w693 -> [w726]
          tunnel: [w720] -> w707 mode=indexing
          n279 = Search 1D Array(1D array=w726, element=w725) -> (index of element=w724:i32)  [unwired: 1 in]
          n280 = Less Than 0?(x=w724) -> (x < 0?=w723:bool)
          n281 = Select(t=0, s=w723, f=1) -> (s? t:f=w720:i32)
        }
        n282 = Sort 1D Array(array=w694) -> (sorted array=w703:string[])
        n283 = Sort 1D Array(array=w693) -> (sorted array=w704:string[])
        n284 = Array Size(array=w693) -> (size(s)=w691:i32)
        n285 = Array Size(array=w694) -> (size(s)=w690:i32)
        n286 = Empty Array?(array=w693) -> (empty?=w706:bool)
        n287 = Equal?(x=w703, y=w704) -> (x = y?=w702:bool)
        n288 = Select(t=enum8{"False", "True", "Mixed"}."True" ("All Files Selection"), s=w702, f=enum8{"False", "True", "Mixed"}."Mixed" ("All Files Selection")) -> (s? t:f=w698:enum8{"False", "True", "Mixed"})
        n289 = property on="Current Branch Changelist" class="MCListbox (strict)"(error in=w708, "ItemSyms"=w707) -> (error out=w692:errorcluster)  [unwired: 1 in, 1 out]
        n290 = Select(t=enum8{"False", "True", "Mixed"}."False" ("All Files Selection"), s=w706, f=w698) -> (s? t:f=w696:enum8{"False", "True", "Mixed"})
        n291 = case "No changelist available?" shown="False" w687 {
          tunnel: w692 -> [w717 w719]
          tunnel: [w716 w719] -> w700
          tunnel: w691 -> [w715 _]
          tunnel: w690 -> [w714 _]
          tunnel: [w713 ""] -> w686
          frame False {
            n292 = Format Into String(format string="%d/%d viewed", error in=w717, w715, w714) -> (resulting string=w713:string, error out=w716:errorcluster)  [unwired: 1 in]
          }
          frame True {
          }
        }
        n293 = property on="All Files Selection" class="MixedCheckbox (strict)"(error in=w700, "Value"=w696, "Text.Text"=w686) -> (error out=w697:errorcluster)  [unwired: 1 in, 1 out]
      }
      frame "Check for LabVIEW File" {
        # "Check if the file for compare is a LabVIEW compare supported file type"
        n294 = Unbundle By Name(w729) -> ("LabVIEW Compare File Extensions"=w735:string[], "File to Compare"=w727:string)
        n295 = String To Path(string=w727) -> (path=w738:path)
        n296 = call <vilib>:"Get File Extension.vi"("error in (no error)"=w734, "file"=w738) -> ("error out"=w733:errorcluster, "lowercase file extension"=w737:string)  [unwired: 5 in, 3 out]
        n297 = Search 1D Array(1D array=w735, element=w737) -> (index of element=w736:i32)  [unwired: 1 in]
        n298 = Less Than 0?(x=w736) -> (x < 0?=w732:bool)
        n299 = case "Unsupported file?" shown="True" w732 {
          tunnel: w733 -> [w740 w747]
          tunnel: w731 -> [_ w746]
          tunnel: [w740 w745] -> w730
          tunnel: w729 -> [w739 w743]
          tunnel: [w739 w742] -> w728
          tunnel: w727 -> [_ w741]
          frame False {
            # "Supported file. No restrictions."
          }
          frame True {
            w751 = "The selected file type is not supported for comparison.\nClick Force Compare to compare anyway or click Open File to open the file instead."  # Message
            w752 = "Unsupported file type for comparison"  # Window Title
            # "Decide whether to force compare or open file or cancel the operation"
            n300 = call <vilib>:"Three Button Dialog.vi"("Window Title (\"\")"=w752, "Right Button Text (\"Cancel\")"="Cancel" ("Right Button Text (\"Cancel\")"), "Center Button Text (\"No\")"="Open File" ("Center Button Text (\"No\")"), "Left Button Text (\"Yes\")"="Force Compare" ("Left Button Text (\"Yes\")"), "message"=w751) -> ("Which Button?"=w744:T9)  [unwired: 6 in]
            n301 = case shown="\"Center Button\"" w744 {
              tunnel: w747 -> [w754 w758 w772]
              tunnel: w746 -> [_ w762 w770]
              tunnel: [w754 w761 w771] -> w745
              tunnel: w743 -> [w753 w757 w769]
              tunnel: [w753 w756 w769] -> w742
              tunnel: w741 -> [_ w755 _]
              frame "Left Button" {
                # "No changes. Continue execution for compare."
              }
              frame "Center Button" {
                # "Clear Compare states and add states for open"
                n302 = Flush Queue(queue=w762, error in (no error)=w758) -> (queue out=w763:refnum<queue>, error out=w759:errorcluster)  [unwired: 1 out]
                n303 = for {
                  tunnel: string[] ["Open File", "Add File to Viewed List", "Update Viewed Status"] -> [w765] mode=indexing
                  shift-right: [w767] -> w761
                  shift-left: w759 -> [w768]
                  shift-right: [w764] -> _
                  shift-left: w763 -> [w766]
                  n304 = Enqueue Element(queue=w766, element=w765, error in (no error)=w768) -> (queue out=w764:refnum<queue>, error out=w767:errorcluster)  [unwired: 1 in, 1 out]
                }
                n305 = Bundle By Name(cluster=w757, "Viewed File"=w755, "File to Open"=w755) -> (w756:T3)
              }
              frame "Right Button", "Window Close" {
                # "Clear Compare states"
                n306 = Flush Queue(queue=w770, error in (no error)=w772) -> (error out=w771:errorcluster)  [unwired: 2 out]
              }
            }
          }
        }
      }
      frame "Open File" {
        # "Open the file in the default application"
        n307 = Unbundle By Name(w778) -> ("Repository Path"=w775:path, "File to Open"=w774:string)
        n308 = Build Path(base path=w775, name or relative path=w774) -> (appended path=w773:path)
        n309 = call <vilib>:"Open a Document on Disk.vi"("error in (no error)"=w777, "document path"=w773) -> ("error out"=w776:errorcluster)  [unwired: 5 in]
      }
      frame "Backup File" {
        w780 = TRUE  # overwrite
        # "Same file with some added suffix"
        # "Move the file to the same location with different file name.\nIt deletes the original file."
        # "Add some suffix to differentiate"
        # "Backup the checked out file as we need to temporarily update it from the other branch/commit"
        n310 = Unbundle By Name(w786) -> ("Repository Path"=w783:path, "File to Compare"=w794:string)
        n311 = Build Path(base path=w783, name or relative path=w794) -> (appended path=w792:path)
        n312 = call <vilib>:"Get File Extension.vi"("error in (no error)"=w789, "file"=w792) -> ("error out"=w788:errorcluster, "filename without extension"=w790:string, "unmodified file extension"=w782:string)  [unwired: 5 in, 2 out]
        n313 = Strip Path(path=w792) -> (stripped path=w791:path)  [unwired: 1 out]
        n314 = Concatenate Strings(w790, " BACKUP" ("string"), "." ("string"), w782) -> (w784:string)
        n315 = Build Path(base path=w791, name or relative path=w784) -> (appended path=w779:path)
        n316 = Move(source path=w792, error in=w788, 9:w780, 10:w779) -> (error out=w793:errorcluster)  [unwired: 1 in, 2 out]
        n317 = Bundle By Name(cluster=w786, "File to Compare (backup)"=w779) -> (w785:T3)
      }
      frame "Checkout Other" {
        w799 = "\""
        # "Checkout will stage the file. So reset the state and make it unstaged. This will still retain any changes made to the file in the HEAD (current) branch."
        # "Path may have space. Add quotes."
        # "Checkout the file from other branch/commit (used to download the file from the other branch/commit)"
        n318 = Unbundle By Name(w805) -> ("Branch/Commit to Compare"=w801:string, "File to Compare"=w800:string, "Git API Object"=w803:refnum<class "GIT-api.lvclass">)
        n319 = Concatenate Strings("-- " ("string"), w799, w800, w799) -> (w795:string)
        n320 = call <vilib>:"GIT-Checkout.vi"("param"=w795, "error in"=w804, "branch name"=w801, "git-api in"=w803) -> ("error out"=w798:errorcluster, "git-api out"=w796:refnum<class "GIT-api.lvclass">)  [unwired: 6 in]
        n321 = call <vilib>:"GIT-Reset.vi"("param"=w795, "error in"=w798, "git-api in"=w796) -> ("error out"=w797:errorcluster)  [unwired: 6 in, 2 out]
      }
      frame "Rename File" {
        w809 = TRUE  # overwrite
        # "Add the file to be deleted later"
        # "Same file with some added suffix"
        # "Move the file to the same location with different file name.\nIt deletes the original file."
        # "Add some suffix to differentiate"
        # "Rename the checked out file which will be later used for compare"
        n322 = Unbundle By Name(w815) -> ("Files to Delete"=w808:path[], "Repository Path"=w812:path, "File to Compare"=w823:string)
        n323 = Build Path(base path=w812, name or relative path=w823) -> (appended path=w821:path)
        n324 = call <vilib>:"Get File Extension.vi"("error in (no error)"=w818, "file"=w821) -> ("error out"=w817:errorcluster, "filename without extension"=w819:string, "unmodified file extension"=w811:string)  [unwired: 5 in, 2 out]
        n325 = Strip Path(path=w821) -> (stripped path=w820:path)  [unwired: 1 out]
        n326 = Concatenate Strings(w819, " TEMP" ("string"), "." ("string"), w811) -> (w813:string)
        n327 = Build Path(base path=w820, name or relative path=w813) -> (appended path=w806:path)
        n328 = Insert Into Array(array=w808, new element=w806) -> (w807:path[])  [unwired: 1 in]
        n329 = Move(source path=w821, error in=w817, 9:w809, 10:w806) -> (error out=w822:errorcluster)  [unwired: 1 in, 2 out]
        n330 = Bundle By Name(cluster=w815, "Files to Delete"=w807, "File to Compare (other)"=w806) -> (w814:T3)
      }
      frame "Restore File" {
        w828 = TRUE  # overwrite
        # "Move the file to the same location with different file name.\nIt deletes the original file."
        # "Restore the file as it was before"
        n331 = Unbundle By Name(w827) -> ("File to Compare (backup)"=w825:path, "Repository Path"=w829:path, "File to Compare"=w831:string)
        n332 = Build Path(base path=w829, name or relative path=w831) -> (appended path=w826:path)
        n333 = Move(source path=w825, error in=w824, 9:w828, 10:w826) -> (error out=w830:errorcluster)  [unwired: 1 in, 2 out]
      }
      frame "Prepare Compare Options" {
        w854 = ""
        # "No 'space' required to be concatenated. It is already included in the flag."
        # "Prepare the command line options for the LabVIEW comparison flags"
        n334 = Unbundle By Name(w835) -> ("LabVIEW Compare Options.VI Attributes"=w853:bool, "LabVIEW Compare Options.Front Panel"=w846:bool, "LabVIEW Compare Options.FP position/size"=w845:bool, "LabVIEW Compare Options.Block Diagram"=w844:bool, "LabVIEW Compare Options.BD cosmetic"=w843:bool, "LabVIEW Compare Options.BD position/size"=w842:bool)
        n335 = Select(t=w854, s=w853, f="-noattr ") -> (s? t:f=w841:string)
        n336 = Select(t=w854, s=w846, f="-nofp ") -> (s? t:f=w840:string)
        n337 = Select(t=w854, s=w845, f="-nofppos ") -> (s? t:f=w839:string)
        n338 = Select(t=w854, s=w844, f="-nobd ") -> (s? t:f=w838:string)
        n339 = Select(t=w854, s=w843, f="-nobdcosm ") -> (s? t:f=w837:string)
        n340 = Select(t=w854, s=w842, f="-nobdpos ") -> (s? t:f=w836:string)
        n341 = Concatenate Strings(w841, w840, w839, w838, w837, w836) -> (w833:string)
        n342 = call <vilib>:"Trim Whitespace.vi"("string"=w833) -> ("trimmed string"=w832:string)  [unwired: 1 in]
        n343 = Bundle By Name(cluster=w835, "LabVIEW Compare Options Command"=w832) -> (w834:T3)
      }
      frame "LabVIEW Compare" {
        w866 = TRUE  # wait until completion?
        # "Other branch file is first to know what changes happened in the current branch"
        # "This should get the correct path from any LabVIEW version this VI runs"
        # "Path may have space. Add quotes."
        # "Perform the comparison"
        n344 = Unbundle By Name(w872) -> ("File to Compare (other)"=w856:path, "Repository Path"=w871:path, "File to Compare"=w870:string, "LabVIEW Compare Options Command"=w858:string)
        n345 = Build Path(base path=w871, name or relative path=w870) -> (appended path=w868:path)
        n346 = VI Library() -> (path=w862:path)
        n347 = Build Path(base path=w862, name or relative path="..\\..\\Shared\\LabVIEW Compare\\LVCompare.exe") -> (appended path=w860:path)
        n348 = Format Into String(format string="\"%s\" \"%s\" \"%s\" %s", error in=w869, w860, w856, w868, w858) -> (resulting string=w864:string, error out=w865:errorcluster)  [unwired: 1 in]
        n349 = call <vilib>:"Trim Whitespace.vi"("string"=w864) -> ("trimmed string"=w857:string)  [unwired: 1 in]
        n350 = Default Directory() -> (w863:path)
        n351 = call <vilib>:"System Exec.vi"("wait until completion? (T)"=w866, "error in (no error)"=w865, "working directory"=w863, "command line"=w857) -> ("error out"=w867:errorcluster)  [unwired: 4 in, 3 out]
      }
      frame "Delete Files" {
        # "The same files may have been compared multiple times and might have tracked to be deleted all those times. So remove the duplicate entries.\nNote: The file 'Move' operation would have overwritten the file if it already existed. So only one file but tracked multiple times."
        # "Delete the files that were introduced by the tool"
        n352 = Unbundle By Name(w877) -> ("Files to Delete"=w876:path[])
        n353 = call-poly <userlib>:"Remove Duplicates from 1D Array__ogtk.vi"("Input Array"=w876) -> ("Output Array"=w873:path[])  [unwired: 1 out]
        n354 = for {
          shift-right: [w880] -> w874
          shift-left: w875 -> [w881]
          tunnel: w873 -> [w878] mode=indexing
          n355 = call-poly <userlib>:"File Exists__ogtk.vi"("file path"=w878) -> ("exists"=w879:bool)  [unwired: 6 in, 1 out]
          n356 = case "File Exists?" shown="True" w879 {
            tunnel: w881 -> [w882 w885]
            tunnel: [w882 w884] -> w880
            tunnel: w878 -> [_ w883]
            frame False {
            }
            frame True {
              n357 = Delete(path (use dialog)=w883, error in=w885) -> (error out=w884:errorcluster)  [unwired: 3 in, 2 out]
            }
          }
        }
      }
      frame "Stop" {
        # "Performs actions when the VI is stopped."
        n358 = for {
          tunnel: string[] ["Delete Files", "Exit"] -> [w892] mode=indexing
          shift-right: [w894] -> w889
          shift-left: w890 -> [w895]
          shift-right: [w891] -> _
          shift-left: w888 -> [w893]
          n359 = Enqueue Element(queue=w893, element=w892, error in (no error)=w895) -> (queue out=w891:refnum<queue>, error out=w894:errorcluster)  [unwired: 1 in, 1 out]
        }
      }
      frame "Exit" {
        w898 = TRUE  # Exit?
        # "Finish the execution"
        n360 = Release Queue(queue=w896, error in (no error)=w900) -> (error out=w897:errorcluster)  [unwired: 1 in, 2 out]
      }
      frame "Error" {
        # "In case of any Git API initialization errors, we need to disable the controls."
        # "Show the error dialog and clear out the operations. Update controls status."
        n361 = call <vilib>:"Simple Error Handler.vi"("error in (no error)"=w908) -> ("error out"=w907:errorcluster)  [unwired: 4 in, 4 out]
        n362 = call <vilib>:"Clear Errors.vi"("error in (no error)"=w907) -> ("error out"=w906:errorcluster)  [unwired: 5 in, 1 out]
        n363 = Flush Queue(queue=w905, error in (no error)=w906) -> (queue out=w902:refnum<queue>, error out=w903:errorcluster)  [unwired: 1 out]
        n364 = for {
          tunnel: string[] ["Enable Disable Controls"] -> [w911] mode=indexing
          shift-right: [w913] -> w901
          shift-left: w903 -> [w914]
          shift-right: [w910] -> _
          shift-left: w902 -> [w912]
          n365 = Enqueue Element(queue=w912, element=w911, error in (no error)=w914) -> (queue out=w910:refnum<queue>, error out=w913:errorcluster)  [unwired: 1 in, 1 out]
        }
      }
    }
  }
  n366 = invoke class="VI" method="FP.Close"(error in=w2) -> (error out=w1:errorcluster)  [unwired: 2 in, 2 out]
  n367 = call <vilib>:"Clear Errors.vi"("error in (no error)"=w1) -> ()  [unwired: 5 in, 2 out]
